vi "Core_Chem_User_Interface_v1.1.vi"() -> ()   [LabVIEW 2014]
uses:
  C:/Program Files (x86)/National Instruments/LabVIEW 2014/examples/Data Communication/Network Streams/Simple Network Streams/support/Network Stream Command.ctl
  <vilib>/dex/Stream Element Allocation Mode.ctl
  <vilib>/Platform/TimedLoop/XDataNode/timing_clust.ctl
  <vilib>/Platform/TimedLoop/XDataNode/nitl_modes.ctl
  <vilib>/Platform/TimedLoop/XDataNode/wakeup.ctl
  <vilib>/Utility/tcp.llb/UDP Multicast Read-Only Open.vi
  <vilib>/platform/TimedLoop/XDataNode/XDataNode.xnode
  <vilib>/Platform/TimedLoop/XDataNode/XDNodeRunTimeDep.lvlib
  <vilib>/FTP/NI_FTP.lvlib
panel:
  in  "Flight Number 2":string
  out "Create folder error out 2":errorcluster
  out "Network to cRIO live status":bool
  out "Create folder error out":errorcluster
  in  "Confirm Flight Number":bool
  out "PRTAFT_UDP_In":string
  out "TWBOZO01":string
  out "CABOZO01":string
  out "TEIOZO01":string
  out "CHTSOO01":string
  out "CHFGGA01":string
  out "AL52CO01":string
  in  "Flight Number":string
  in  "Tab Control":T1(tab)
  out "MFM":dbl(graph)
  out "PRTAFT_DLU":string
  in  "name":string="239.1.4.6"
  in  "Port":u16=50001
  out "FGGA":string
  out "CO":string
  out "Ozone":string
  out "Cabin Ozone":string
  out "Ambient Ozone":string
  out "SO2":string
  out "Raw Signal (Hz)":dbl(graph)
  out "CO Concentration":dbl(graph)
  out "Fluorsecence Cell Pressure":dbl(graph)
  out "Monochromater Flow":dbl(graph)
  out "Lamp Flow Controller":dbl(graph)
  in  "CO UDP Time Offset":i32=1
  out "CO2 Pressure\nDelivery (PSIA)":dbl(slide) scale=0.0..100.0
  out "CO CAL Status":bool
  out "Std\nContent (barG)":dbl(slide) scale=0.0..220.0
  out "N2\nContent (barG)":dbl(slide) scale=0.0..220.0
  out "CO2\nContent (barG)":dbl(slide) scale=0.0..170.0
  in  "CO CAL":bool
  in  "CO Vacuum (eV7)":bool
  out "CO Event error out":errorcluster
  out "CO command sender error out":errorcluster
  out "CO Zero":T2(array[cluster])
  out "CO Sensitivity":T3(array[cluster])
  in  "Ozone V6":bool
  out "TEI49C Sample Flow B":dbl(graph)
  out "TEi49C Concentration":dbl(graph)
  out "TEI49C Sample Flow A":dbl(graph)
  out "Ozone Event error out":errorcluster
  out "Ozone command sender error out":errorcluster
  out "Ozone Zeroing\nTime Remain (sec)":u32
  in  "Ozone Zeroing":bool
  in  "Ozone UDP Time Offset":i32=1
  in  "FGGA Pump":bool
  in  "FGGA Shutdown":bool
  in  "V1":bool
  in  "V2":bool
  in  "MFC_1\nSLPM Value":dbl
  in  "V3":bool
  in  "V4":bool
  in  "FGGA Restart":bool
  out "MFC1 Cal Flow":dbl(graph)
  out "Cell temperature":dbl(graph)
  out "Cell pressure":dbl(graph)
  out "CO2 Dry":dbl(graph)
  out "CH4 Dry":dbl(graph)
  out "H2O":dbl(graph)
  out "CO2":dbl(graph)
  out "CH4":dbl(graph)
  in  "Flush High Tank":bool
  in  "Flush Low Tank":bool
  in  "Flush Target Tank":bool
  out "Flush High Tank\nTime Remain (sec)":u32
  out "Flush Low Tank\nTime Remain (sec)":u32
  out "Flush Target Tank\nTime Remain (sec)":u32
  in  "High Cal":bool
  out "High Cal\nFlush Time Remain (sec)":u32
  out "High Cal\nCal Time Remain (sec)":u32
  in  "Low Cal":bool
  in  "Target Cal":bool
  in  "Span Cal Synchronise with\nCO":bool
  out "Low Cal\nFlush Time Remain (sec)":u32
  out "Low Cal\nCal Time Remain (sec)":u32
  out "Target Cal\nFlush Time Remain (sec)":u32
  out "Target Cal\nCal Time Remain (sec)":u32
  in  "MFC_1 User Set Value":dbl=3.0
  out "FGGA command sender error out":errorcluster
  out "FGGA Event Error out":errorcluster
  in  "FGGA UDP Time Offset":i32=1
  in  "FGGA pump\nsync to WoW":bool
  out "WoW Flag":string="0"
  in  "Inst_alm_thresh":i32=220
  in  "3hr_alm_thresh":i32=80
  in  "Simulate Inst Conc":i32
  in  "Simulate 3hr Average Conc":dbl
  in  "Simulate 2B Conc":bool
  out "2B Ozone concentration":dbl(graph)
  out "2B Ozone flow rate":dbl(graph)
  out "2BOzone Event error out":errorcluster
  out "2BOzone command sender error out":errorcluster
  in  "Ambient = OFF\nCabin = ON":bool
  in  "V9":bool
  in  "V8":bool
  in  "SO2 V6":bool
  in  "MFC_2\nSLPM Value":dbl
  in  "MFC_3\nSLPM Value":dbl=2.0
  in  "Simulate STEL Conc":dbl
  in  "Simulate TWA Conc":dbl
  in  "SO2 Offset":dbl
  in  "SO2 Slope":dbl=1.0
  in  "10mins STEL Limit":i32=700
  in  "8hr TWA Limit":i32=490
  in  "Simulate Conc":bool
  out "TEI43i MFC2 Cal Flow":dbl(graph)
  out "TEI43i MFC3 Sample Flow":dbl(graph)
  out "TEi43C Concentration":dbl(graph)
  out "TEI43C Sample Flow":dbl(graph)
  out "SO2 Event error out":errorcluster
  out "SO2 command sender error out":errorcluster
  in  "SO2 Flush":bool
  in  "SO2 CAL":bool
  in  "MFC_2 User Set Value":dbl=2.5
  in  "MFC_3 User Set Value":dbl=2.0
  out "SO2 Flush\nTime Remain (sec)":u32
  in  "SO2 Zeroing":bool
  out "SO2 Zeroing\nTime Remain (sec)":u32
  out "SO2 CAL\nTime Remain (sec)":u32
  in  "SO2 UDP Time Offset":i32=1
  in  "cRIO File IO Stop\n(USB Flash Drive Unmount)":bool
  in  "FTP ASCII Files to Local":bool
  in  "Transfer FGGA Files":bool
  out "File List":string[](array[string])
  out "FGGA File Transfer Error out":errorcluster
  out "Move to FM Error out":errorcluster
  out "USB Disk Space Used %":dbl(slide) scale=0.0..100.0
  out "PTP Sync":bool
  out "CPU Total %":dbl(graph)
  # "conc\ncounts\nsens\nzero\nlampflow\nlamptemp\nmonoflow\nmonotemp\nmonopress\ncellpress\ncalpress\ntemppmt\ncalconc\nerr\ncal_counter\nerr_counter\nCO_vacuum_status\nIn_Cal\nALEG1_press_delivery\nALREG1_press_content\nALREG2_press_content\nALREG3_press_content"
  # "concentration\npmt_volt\nlamp_volt\nlamp_intens\ninternal_temper\nreact_temper\nreact_press\nflow\nflags\nten_min_so2\neight_hr_so2\nten_min_so2_alm\neight_hr_so2_alm\nMFC_2absolute_pressure\nMFC_2temperature\nMFC_2volumetic_flow\nMFC_2mass_flow\nMFC_2set_point\nMFC_3_absolute_pressure\nMFC_3_temperature\nMFC_3volumetic_flow\nMFC_3mass_flow\nMFC_3set_point\nV6\nV8\nV9\nMFC2_Set_Value\nMFC3_Set_Value"
  # "ch4\nco2\nh2o\npress_torr\ntemp_c\nfit_flag\nrda_usec\nrdb_usec\nch4_dry\nco2_dry\nMFC_1_absolute_pressure\nMFC_1_temperature\nMFC_1volumetic_flow\nMFC_1mass_flow\nMFC_1set_point\nV1\nV2\nV3\nV4\nrestart_FGGA\nFGGA_Pump\nCAL_MFC_1Set_Value"
  # "conc\ntemp\npress\nflow"
  # "conc\ntemp\npress\nflow\nthreehr_oz\nInst_alarm\nthreehr_alarm"
  # "conc\nbenchtemp\npress\ncellAint\ncellBint\nFlowA\nFlowB\nlamptemp\nflag\nV6"
  # "DIRECT CONTROL"
  # "DIRECT CONTROLS"
  # "DIRECT CONTROLS"
  # "TEi43c"
  # "TEi43i"
  # "DIRECT CONTROLS"
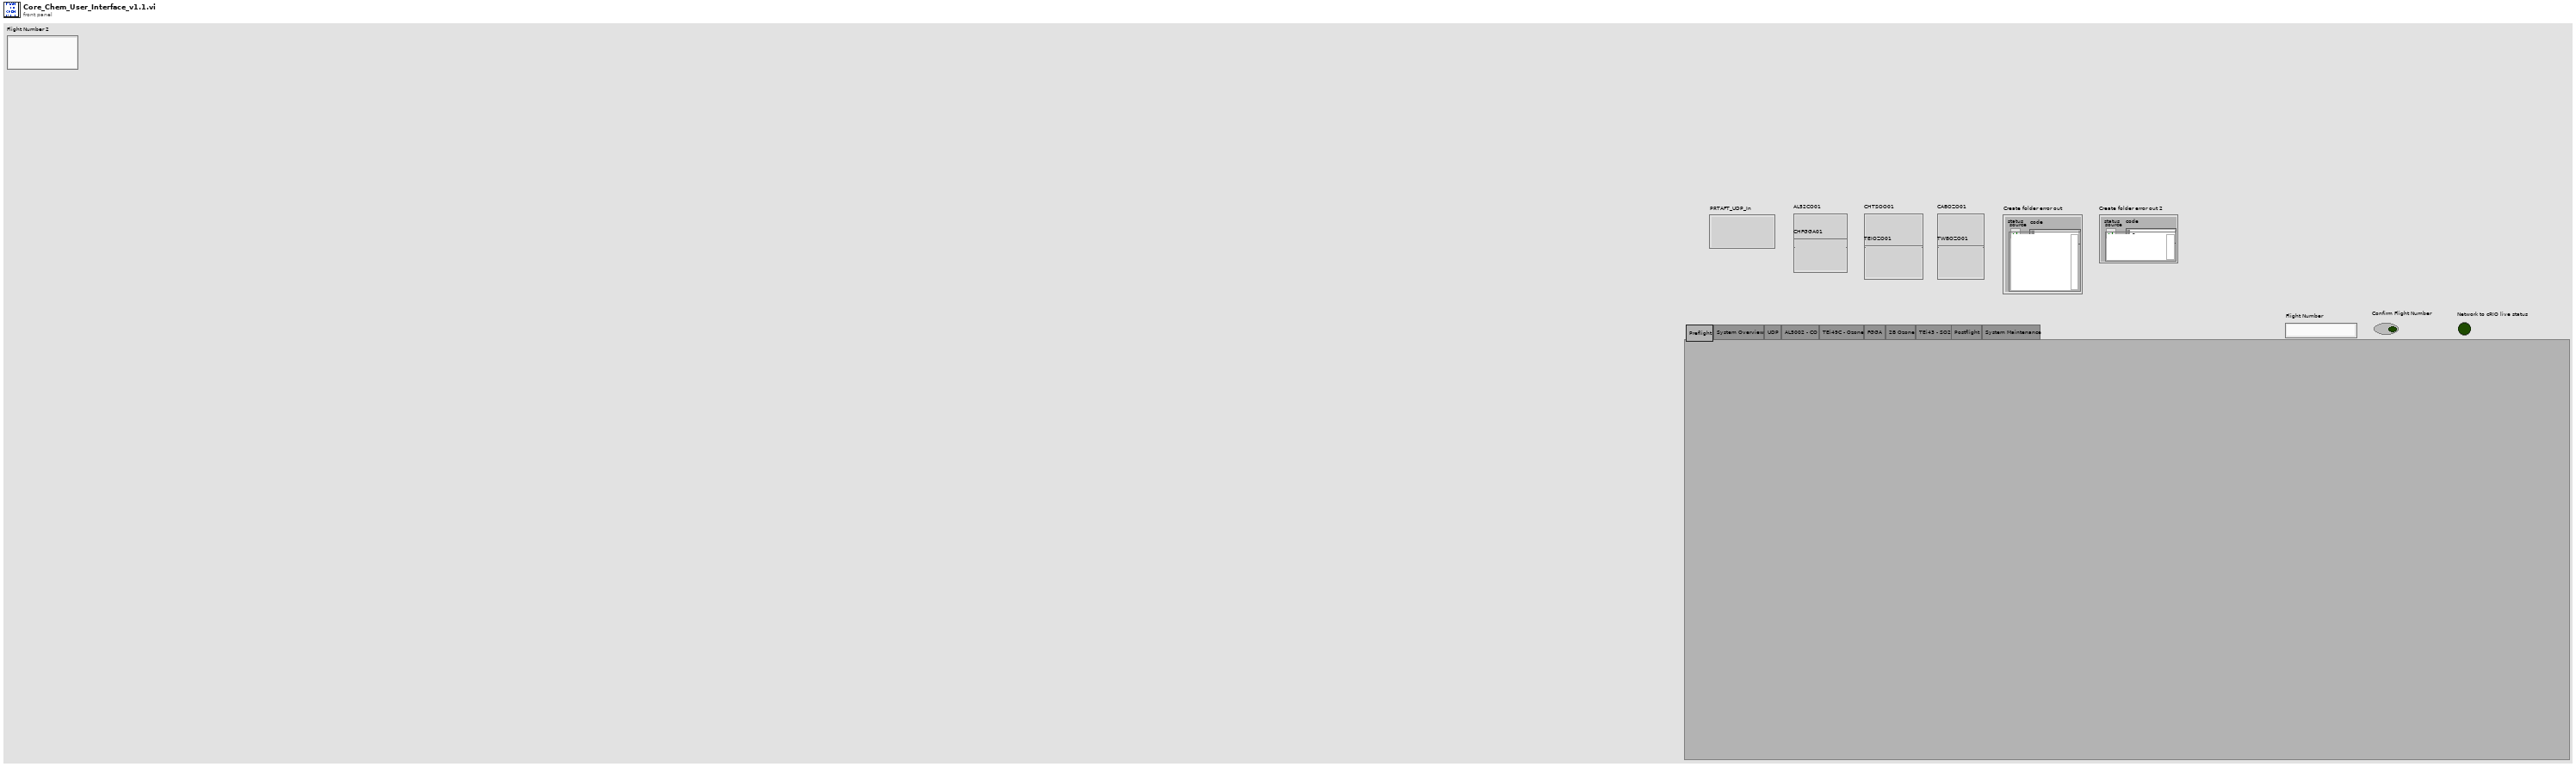
[diagram p1: front panel]
types:
  T1 = enum32{"Preflight", "System Overview", "UDP", "AL5002 - CO", "TEi49C - Ozone", "FGGA", "2B Ozone", "TEi43 - SO2", "Postflight", "System Maintenance"}
  T2 = cluster{"time stamp":timestamp, "CO Offset":dbl}[]
  T3 = cluster{"time stamp":timestamp, "CO Sensitivity":dbl}[]
  T4 = typedef "Network Stream Command.ctl" = cluster{"Message":string, "Message Data":variant}
  T5 = typedef "Stream Element Allocation Mode.ctl" = u32
  T6 = typedef "XDNodeRunTimeDep.lvlib/timing_clust.ctl" = cluster{"Expected End [f-1]":u64, "Actual End [f-1]":u64, "Finished Late? [f-1]":bool, "Expected End [i-1]":u64, "Actual End [i-1]":u64, "Finished Late? [i-1]":bool, "Expected Start [i]":u64, "Actual Start [i]":u64, "Expected Start [f]":u64, "Actual Start [f]":u64, "Source Name":string, "Structure Name":string, "Period":i64, "Deadline":i64, "Offset":i64, "Start":i64, "Priority":i32, "Timeout":i32, "Mode":T7, "Wakeup Reason":T8, "Error":errorcluster, "Source Type":string, "Secondary Source Type":string, "Global End Time":u64, "Global Start Time":u64, "Frame Duration":u64, "Iteration Duration":u64, "Assigned CPU":i32, "I/O Scan Engine Mode":u32}
  T7 = typedef "XDNodeRunTimeDep.lvlib/nitl_modes.ctl" = enum32{"No Change", "Process missed periods, maintain original phase", "Discard missed periods, maintain original phase", "Process missed periods, ignore original phase", "Discard missed periods, ignore original phase"}
  T8 = typedef "XDNodeRunTimeDep.lvlib/wakeup.ctl" = enum32{"Normal", "Aborted", "Asynchronous wakeup", "Timing source error", "Timed loop error", "Timeout"}
  T9 = typedef "NI_FTP.lvlib/FTP Session.ctl" = refnum<k5>
  T10 = typedef "NI_FTP.lvlib/FTP File Info.ctl" = cluster{"type":enum16{"unknown", "file", "dir", "link"}, "permissions":string, "owner":string, "group":string, "size":i32, "date":string, "name":string, "link name":string}
  T11 = cluster{"Message":string, "Message 2":string, "Message 3":string}
  T12 = cluster{"Message":string, "Message 2":string, "Message 3":string, "Message 4":string}
  T13 = cluster{"Message":string, "Message 3":string, "Message 4":string}
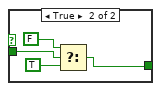
[diagram p8: hidden frame]
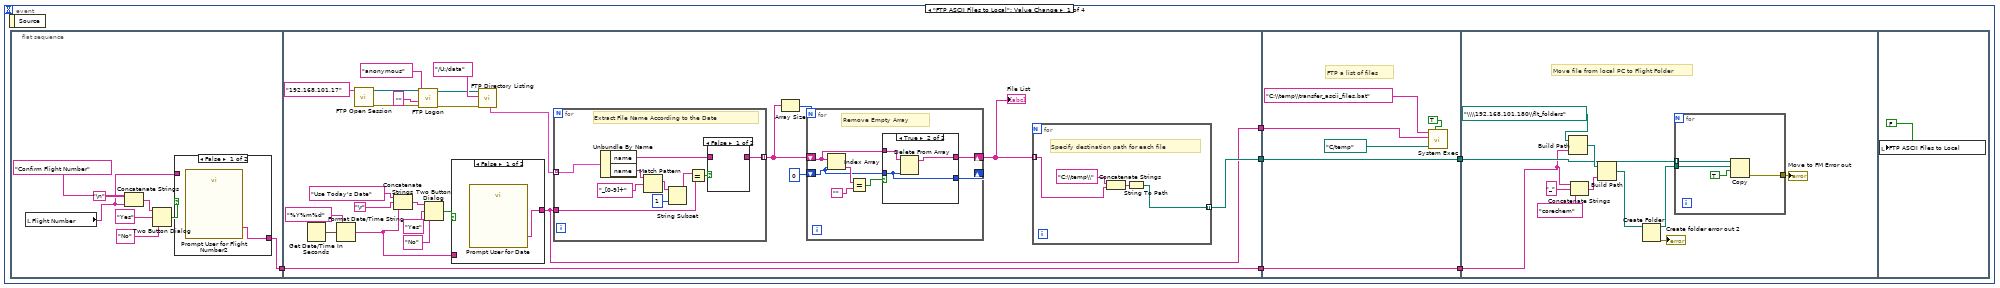
[diagram p11: hidden frame]
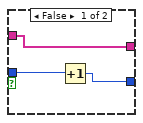
[diagram p14: hidden frame]
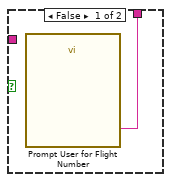
[diagram p16: hidden frame]
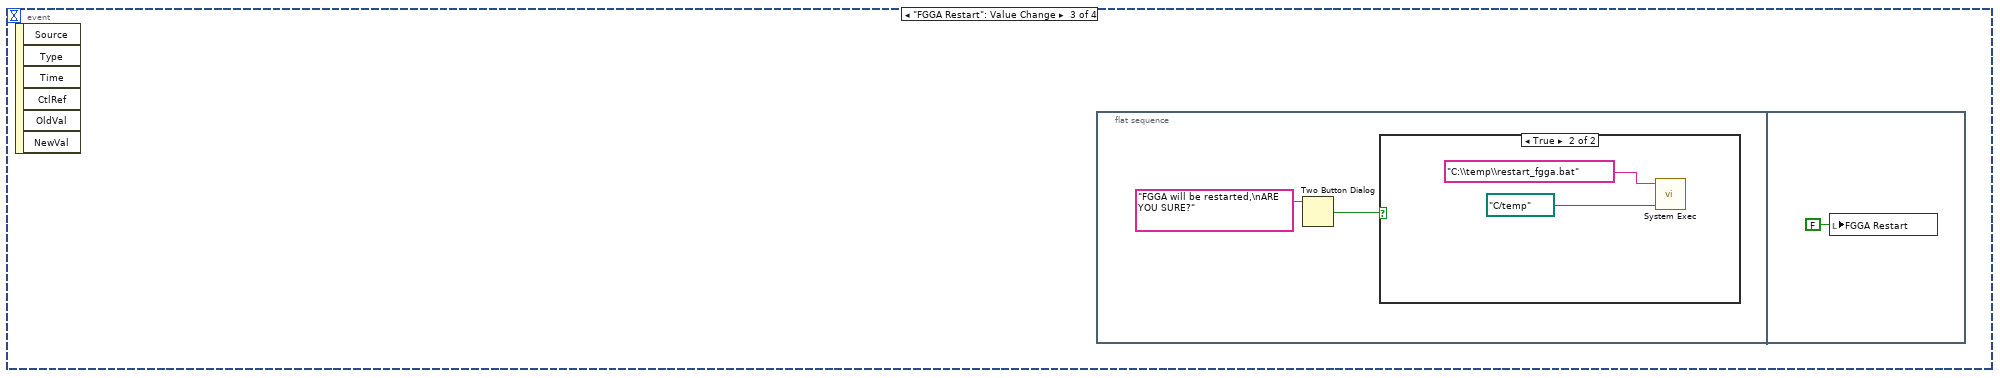
[diagram p18: hidden frame]
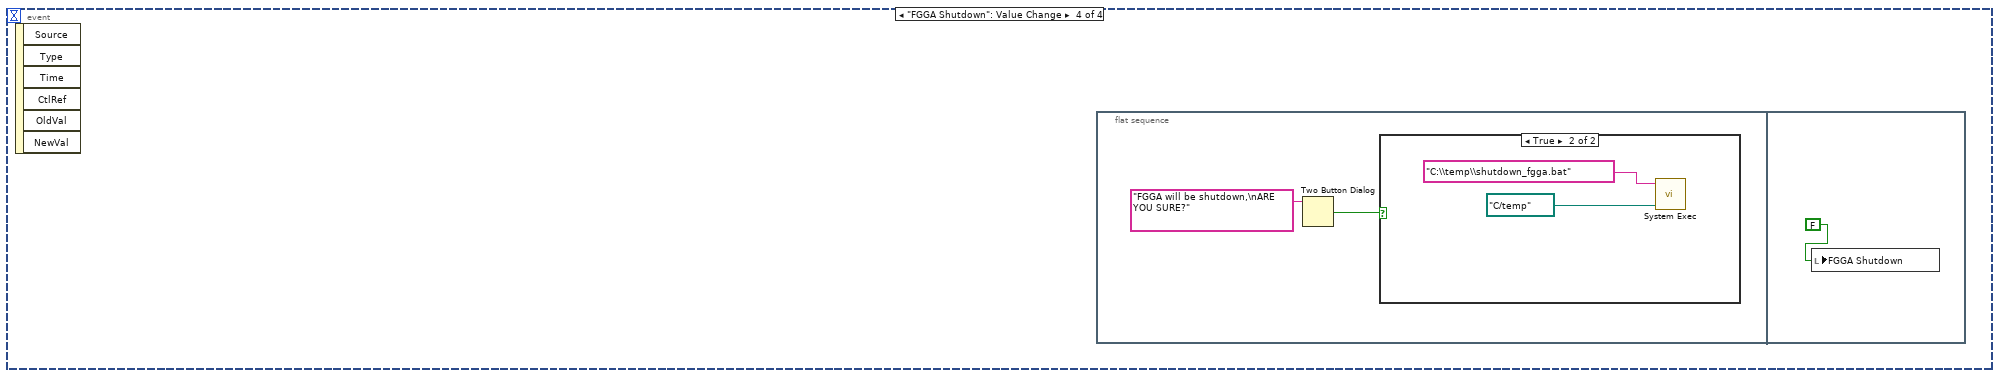
[diagram p20: hidden frame]
diagram:
  w4 = "XXXX"
  w7 = 0
  w8 = 0.0
  w14 = T4 {"Message"="", "Message Data"=variant} ("Message Cluster")
  w20 = T5 0 items=["allocate as needed", "pre-allocate"] ("element allocation mode")
  w26 = T4 {"Message"="", "Message Data"=variant} ("Message Cluster")
  w32 = T5 0 items=["allocate as needed", "pre-allocate"] ("element allocation mode")
  w37 = T4 {"Message"="", "Message Data"=variant} ("Message Cluster")
  w43 = T5 0 items=["allocate as needed", "pre-allocate"] ("element allocation mode")
  w53 = T5 0 items=["allocate as needed", "pre-allocate"] ("element allocation mode")
  w55 = T4 {"Message"="", "Message Data"=variant} ("Message Cluster")
  w62 = T5 0 items=["allocate as needed", "pre-allocate"] ("element allocation mode")
  w64 = T4 {"Message"="", "Message Data"=variant} ("Message Cluster")
  n1 = local write "cRIO File IO Stop\n(USB Flash Drive Unmount)"(FALSE ("Stop File Write")) -> ()
  n2 = local write "Flight Number"(w4) -> ()
  n3 = while {
    shift-right: [w68] -> _
    shift-left: w4 -> [w67]
    stop <- FALSE stop-if-true
    n4 = Not Equal?(x=w67, y="Flight Number") -> (x != y?=w70:bool)
    n5 = case shown="True" w70 {
      tunnel: [w73 w74] -> w68
      tunnel: "Flight Number" -> [_ w74]
      tunnel: w67 -> [w73 _]
      frame False {
      }
      frame True {
        n6 = One Button Dialog(message="Flight Number changed,\nPress flight number button to confirm") -> ()  [unwired: 1 in, 1 out]
      }
    }
    n7 = Wait (ms)(milliseconds to wait=u32 1000) -> ()  [unwired: 1 out]
  }
  n8 = while {
    stop <- FALSE stop-if-true
    # "UDP Read"
    n9 = String To IP(1:"name") -> (0:w81:u32)
    n10 = call-poly <vilib>:"UDP Multicast Open.vi"("multicast addr"=w81, "port"="Port") -> ("error out"=w79:errorcluster, "connection ID"=w78:refnum<k16>)  [unwired: 7 in, 1 out]
    n11 = Wait (ms)(milliseconds to wait=u32 1000) -> ()  [unwired: 1 out]
    n12 = case shown="No Error" w79 {
      selector: w79 -> [w85 _]
      tunnel: w78 -> [w84 _]
      frame No Error {
        w83 = ""
        n13 = while {
          tunnel: w85 -> [w131]
          tunnel: w84 -> [w130]
          shift-right: [w126] -> _
          shift-left: w83 -> [w127]
          shift-right: [w117] -> _
          shift-left: w83 -> [w119]
          shift-right: [w111] -> _
          shift-left: w83 -> [w113]
          shift-right: [w105] -> _
          shift-left: w83 -> [w106]
          shift-right: [w99] -> _
          shift-left: w83 -> [w100]
          shift-right: [w93] -> _
          shift-left: w83 -> [w94]
          shift-right: [w88] -> _
          shift-left: w83 -> [w89]
          stop <- w129 stop-if-true
          n14 = UDP Read(connection ID=w130, 8:w131) -> (data out=w86:string, error out=w129:errorcluster)  [unwired: 2 in, 3 out]
          n15 = Match Pattern(string=w86, regular expression="$TEIOZO01,") -> (match substring=w125:string, after substring=w124:string)  [unwired: 1 in, 2 out]
          n16 = Match Pattern(string=w86, regular expression="$TWBOZO01,") -> (match substring=w103:string, after substring=w102:string)  [unwired: 1 in, 2 out]
          n17 = Match Pattern(string=w86, regular expression="$CABOZO01,") -> (match substring=w109:string, after substring=w108:string)  [unwired: 1 in, 2 out]
          n18 = Match Pattern(string=w86, regular expression="$CHTSOO01,") -> (match substring=w97:string, after substring=w96:string)  [unwired: 1 in, 2 out]
          n19 = Match Pattern(string=w86, regular expression="$CHFGGA01,") -> (match substring=w121:string, after substring=w120:string)  [unwired: 1 in, 2 out]
          n20 = Match Pattern(string=w86, regular expression="$AL52CO01,") -> (match substring=w115:string, after substring=w114:string)  [unwired: 1 in, 2 out]
          n21 = Match Pattern(string=w86, regular expression="$PRTAFT01,") -> (match substring=w92:string, after substring=w91:string)  [unwired: 1 in, 2 out]
          n22 = Concatenate Strings(w125, w124) -> (w123:string)
          n23 = Concatenate Strings(w103, w102) -> (w101:string)
          n24 = Concatenate Strings(w109, w108) -> (w107:string)
          n25 = Concatenate Strings(w97, w96) -> (w95:string)
          n26 = Concatenate Strings(w121, w120) -> (w118:string)
          n27 = Concatenate Strings(w115, w114) -> (w112:string)
          n28 = Concatenate Strings(w92, w91) -> (w87:string)
          n29 = Replace Substring(4:w101, 5:w100) -> (1:w99:string)  [unwired: 2 in, 1 out]
          "TWBOZO01" <- w99
          n30 = Replace Substring(4:w123, 5:w127) -> (1:w126:string)  [unwired: 2 in, 1 out]
          "TEIOZO01" <- w126
          n31 = Replace Substring(4:w107, 5:w106) -> (1:w105:string)  [unwired: 2 in, 1 out]
          "CABOZO01" <- w105
          n32 = Replace Substring(4:w95, 5:w94) -> (1:w93:string)  [unwired: 2 in, 1 out]
          "CHTSOO01" <- w93
          n33 = Replace Substring(4:w87, 5:w89) -> (1:w88:string)  [unwired: 2 in, 1 out]
          "PRTAFT_UDP_In" <- w88
          n34 = Replace Substring(4:w112, 5:w113) -> (1:w111:string)  [unwired: 2 in, 1 out]
          "AL52CO01" <- w111
          n35 = Replace Substring(4:w118, 5:w119) -> (1:w117:string)  [unwired: 2 in, 1 out]
          "CHFGGA01" <- w117
        }
      }
      frame Error {
      }
    }
  }
  n36 = Obtain Queue(name (unnamed)="CO_Command", element data type=w64) -> (queue out=w13:refnum<queue>, error out=w58:errorcluster)  [unwired: 3 in, 1 out]
  n37 = Create Network Stream Writer Endpoint(6:w62, 7:10 ("writer buffer size"), 9:w64, 10:"//192.168.101.17/command/reader/CO" ("reader url"), 11:"/command/writer/CO" ("writer name")) -> (0:w61:errorcluster, 3:w60:refnum<k21>)  [unwired: 2 in]
  n38 = while {
    tunnel: w13 -> [w135]
    tunnel: w58 -> [w134]
    tunnel: [w132] -> _
    stop <- FALSE stop-if-true
    # "CO UI Event Handler Loop"
    n39 = event shown="[4] \"Confirm Flight Number\": Value Change" {
      selector: _ -> [_ _ _ _ _]
      dyn-events: _ -> [_ _ _ _ _]
      timeout: _ -> [_ _ _ _ _]
      tunnel: w135 -> [w142 w149 w153 w160 w167]
      tunnel: w134 -> [w141 w148 w152 w159 w166]
      tunnel: [w136 w143 w151 w158 w165] -> w132
      event "CO CAL": Value Change {
        n40 = event-data() -> ("NewVal"=w139:bool)  [unwired: 1 in]
        n41 = Bundle(cluster=T4 {"Message"="", "Message Data"=variant} ("Message Cluster"), "Message"="CO CAL", "Message Data"=w139) -> (w137:T4)
        n42 = Enqueue Element(queue=w142, element=w137, error in (no error)=w141) -> (error out=w136:errorcluster)  [unwired: 1 in, 2 out]
      }
      event "CO UDP Time Offset": Value Change {
        n43 = event-data() -> ("NewVal"=w146:i32)  [unwired: 1 in]
        n44 = Bundle(cluster=T4 {"Message"="", "Message Data"=variant} ("Message Cluster"), "Message"="UDP Time Offset", "Message Data"=w146) -> (w144:T4)
        n45 = Enqueue Element(queue=w149, element=w144, error in (no error)=w148) -> (error out=w143:errorcluster)  [unwired: 1 in, 2 out]
      }
      event "CO Vacuum (eV7)": Value Change {
        n46 = event-data() -> ("NewVal"=w150:bool)  [unwired: 1 in]
        n47 = Bundle(cluster=T4 {"Message"="", "Message Data"=variant} ("Message Cluster"), "Message"="CO Vacuum", "Message Data"=w150) -> (w154:T4)
        n48 = Enqueue Element(queue=w153, element=w154, error in (no error)=w152) -> (error out=w151:errorcluster)  [unwired: 1 in, 2 out]
      }
      event "cRIO File IO Stop\n(USB Flash Drive Unmount)": Value Change {
        n49 = event-data() -> ("NewVal"=w157:bool)  [unwired: 1 in]
        n50 = Bundle(cluster=T4 {"Message"="", "Message Data"=variant} ("Message Cluster"), "Message"="Stop File Write", "Message Data"=w157) -> (w161:T4)
        n51 = Enqueue Element(queue=w160, element=w161, error in (no error)=w159) -> (error out=w158:errorcluster)  [unwired: 1 in, 2 out]
      }
      event "Confirm Flight Number": Value Change {
        n52 = event-data() -> ()  [unwired: 1 in, 1 out]
        n53 = local read "Flight Number"() -> (w164:string)
        n54 = Bundle(cluster=T4 {"Message"="", "Message Data"=variant} ("Message Cluster"), "Message"="Flight Number", "Message Data"=w164) -> (w168:T4)
        n55 = Enqueue Element(queue=w167, element=w168, error in (no error)=w166) -> (error out=w165:errorcluster)  [unwired: 1 in, 2 out]
      }
    }
    "CO Event error out" <- w132
  }
  n56 = while {
    tunnel: w13 -> [w178]
    shift-right: [w173] -> _
    shift-left: w60 -> [w175]
    shift-right: [w171] -> w49
    shift-left: w61 -> [w177]
    tunnel: w58 -> [w172]
    stop <- w171 stop-if-true
    # "CO UI Command Sender"
    n57 = Dequeue Element(queue=w178, error in (no error)=w172) -> (element=w174:T4)  [unwired: 1 in, 3 out]
    n58 = Unbundle By Name(w174) -> ("Message"=w176:string)
    n59 = case shown="\"UDP Time Offset\"" w176 {
      tunnel: w177 -> [w179 w183 w190 w197 w204 w211]
      tunnel: w175 -> [w180 w186 w193 w200 w207 w214]
      tunnel: w174 -> [_ w185 w192 w199 w206 w213]
      tunnel: [w179 w182 w189 w196 w203 w210] -> w171
      tunnel: [w180 w181 w188 w195 w202 w209] -> w173
      frame "False", Default {
      }
      frame "CO CAL" {
        n60 = shared-variable-write(w186, w183, w185) -> (w184:refnum<k21>, w187:errorcluster)  [unwired: 1 in, 1 out]
        n61 = Flush Stream(8:w187, 11:w184) -> (0:w182:errorcluster, 3:w181:refnum<k21>)  [unwired: 2 in, 1 out]
      }
      frame "UDP Time Offset" {
        n62 = shared-variable-write(w193, w190, w192) -> (w191:refnum<k21>, w194:errorcluster)  [unwired: 1 in, 1 out]
        n63 = Flush Stream(8:w194, 11:w191) -> (0:w189:errorcluster, 3:w188:refnum<k21>)  [unwired: 2 in, 1 out]
      }
      frame "Stop File Write" {
        n64 = shared-variable-write(w200, w197, w199) -> (w198:refnum<k21>, w201:errorcluster)  [unwired: 1 in, 1 out]
        n65 = Flush Stream(8:w201, 11:w198) -> (0:w196:errorcluster, 3:w195:refnum<k21>)  [unwired: 2 in, 1 out]
      }
      frame "Flight Number" {
        n66 = shared-variable-write(w207, w204, w206) -> (w205:refnum<k21>, w208:errorcluster)  [unwired: 1 in, 1 out]
        n67 = Flush Stream(8:w208, 11:w205) -> (0:w203:errorcluster, 3:w202:refnum<k21>)  [unwired: 2 in, 1 out]
      }
      frame "CO Vacuum" {
        n68 = shared-variable-write(w214, w211, w213) -> (w212:refnum<k21>, w215:errorcluster)  [unwired: 1 in, 1 out]
        n69 = Flush Stream(8:w215, 11:w212) -> (0:w210:errorcluster, 3:w209:refnum<k21>)  [unwired: 2 in, 1 out]
      }
    }
  }
  "CO command sender error out" <- w49
  n70 = node-c288() -> (w12:T6)  [unwired: 4 in]
  n71 = Initialize Array(cluster{"time stamp":timestamp, "Y":dbl} {"time stamp"=timestamp(0 s since 1904-01-01), "Y"=0.0}, 30 ("dimension size")) -> (w9:cluster{"time stamp":timestamp, "Y":dbl}[])
  n72 = timed-loop {
    timing: w12 -> [_]
    timing-out: [_] -> w11
    stop <- _ stop-if-true
    # "PC Tasks"
    n73 = node-c288() -> ()  [unwired: 1 in, 1 out]
    n74 = event shown="[1] \"Transfer FGGA Files\": Value Change" {
      selector: _ -> [_ _ _ _]
      dyn-events: _ -> [_ _ _ _]
      timeout: _ -> [_ _ _ _]
      event "FTP ASCII Files to Local": Value Change {
        n75 = event-data() -> ()  [unwired: 1 in, 1 out]
        n76 = flat-sequence {
          tunnel: [w224] -> w218
          tunnel: [w236] -> w223
          tunnel: [w235] -> w221
          tunnel: [w234] -> w219
          tunnel: w218 -> [w234]
          tunnel: w223 -> [w294]
          tunnel: [w294] -> w222
          tunnel: w221 -> [w290]
          tunnel: [w289] -> w220
          tunnel: w219 -> [w289]
          tunnel: w222 -> [w300]
          tunnel: w220 -> [w295]
          frame #0 {
            n77 = local read "Flight Number"() -> (w225:string)
            n78 = Concatenate Strings("Confirm Flight Number" ("message"), "\n", w225) -> (w230:string)
            n79 = Two Button Dialog(message=w230, 1:"No" ("F button name (\"Cancel\")"), 2:"Yes" ("T button name (\"OK\")")) -> (T button?=w226:bool)
            n80 = case shown="False" w226 {
              tunnel: w225 -> [_ w233]
              tunnel: [w232 w233] -> w224
              frame False {
                n81 = call "Prompt User for Flight Number2"() -> ("Flight Number BXXX"=w232:string)  [unwired: 17 in, 2 out]
              }
              frame True {
              }
            }
          }
          frame #1 {
            n82 = Get Date/Time In Seconds() -> (seconds since 1Jan1904=w240:timestamp)
            n83 = Format Date/Time String(time format string (%c)="%Y%m%d", seconds (now)=w240) -> (date/time string=w238:string)  [unwired: 1 in]
            n84 = call <vilib>:"FTP Open Session.vi"("address"="192.168.101.17") -> ("error out"=w255:errorcluster, "ftp session"=w256:T9)  [unwired: 7 in, 2 out]
            n85 = Concatenate Strings("Use Today's Date" ("message"), "\r", w238) -> (w244:string)
            n86 = call <vilib>:"FTP Logon.vi"("error in (no error)"=w255, "password"="", "user"="anonymous", "ftp session"=w256) -> ("error out"=w252:errorcluster, "ftp session out"=w251:T9)  [unwired: 4 in, 2 out]
            n87 = Two Button Dialog(message=w244, 1:"No" ("F button name (\"Cancel\")"), 2:"Yes" ("T button name (\"OK\")")) -> (T button?=w241:bool)
            n88 = case shown="False" w241 {
              tunnel: [w259 w260] -> w235
              tunnel: w238 -> [_ w260]
              frame False {
                n89 = call "Prompt User for Date"() -> ("Date"=w259:string)  [unwired: 17 in, 2 out]
              }
              frame True {
              }
            }
            n90 = call <vilib>:"FTP Directory Listing.vi"("error in (no error)"=w252, "directory path"="/U:/data", "ftp session"=w251) -> ("dir list"=w250:T10[])  [unwired: 4 in, 4 out]
            n91 = for {
              tunnel: w250 -> [w280] mode=indexing
              tunnel: [w279] -> w247 mode=indexing
              tunnel: w235 -> [w278]
              # "Extract File Name According to the Date"
              n92 = Unbundle By Name(w280) -> ("name"=w286:string, "name"=w285:string)
              n93 = Match Pattern(string=w285, regular expression="_[0-9]+") -> (match substring=w283:string)  [unwired: 1 in, 3 out]
              n94 = String Subset(string=w283, offset (0)=1) -> (substring=w281:string)  [unwired: 1 in]
              n95 = Equal?(x=w281, y=w278) -> (x = y?=w287:bool)
              n96 = case shown="False" w287 {
                tunnel: w286 -> [_ w288]
                tunnel: [_ w288] -> w279
                frame False {
                }
                frame True {
                }
              }
            }
            n97 = Array Size(array=w247) -> (size(s)=w249:i32)
            n98 = for {
              N: w249 -> [_]
              shift-right: [w267] -> w237
              shift-left: w247 -> [w268]
              shift-right: [w265] -> _
              shift-left: 0 -> [w266]
              # "Remove Empty Array"
              n99 = Index Array(array=w268, index=w266) -> (element=w270:string)
              n100 = Equal?(x=w270, y="") -> (x = y?=w269:bool)
              n101 = case shown="True" w269 {
                tunnel: w268 -> [w274 w277]
                tunnel: w266 -> [w273 w275]
                tunnel: [w274 w276] -> w267
                tunnel: [w272 w275] -> w265
                frame False {
                  n102 = Increment(x=w273) -> (x+1=w272:i32)
                }
                frame True {
                  n103 = Delete From Array(array=w277, index=w275) -> (array with subset deleted=w276:string[])  [unwired: 1 in, 1 out]
                }
              }
            }
            "File List" <- w237
            n104 = for {
              tunnel: w237 -> [w263] mode=indexing
              tunnel: [w261] -> w236 mode=indexing
              # "Specify destination path for each file"
              n105 = Concatenate Strings("C:\\temp\\", w263) -> (w262:string)
              n106 = String To Path(string=w262) -> (path=w261:path)
            }
          }
          frame #2 {
            # "FTP a list of files"
            n107 = call <vilib>:"System Exec.vi"("wait until completion? (T)"=TRUE, "working directory"=path "C:/temp", "standard input"=w290, "command line"="C:\\temp\\transfer_ascii_files.bat") -> ()  [unwired: 4 in, 4 out]
          }
          frame #3 {
            # "Move file from local PC to Flight Folder"
            n108 = Build Path(base path=path "\\\\192.168.101.180\\flt_folders" ("path"), name or relative path=w295) -> (appended path=w302:path)
            n109 = Concatenate Strings(w295, "_" ("string"), "corechem" ("string")) -> (w301:string)
            n110 = Build Path(base path=w302, name or relative path=w301) -> (appended path=w297:path)
            n111 = Create Folder(path (use dialog)=w297) -> (created path=w296:path, error out=→"Create folder error out 2":errorcluster)  [unwired: 2 in, 1 out]
            n112 = for {
              tunnel: w296 -> [w309]
              tunnel: [w308] -> w299
              tunnel: w300 -> [w306] mode=indexing
              n113 = Copy(9:TRUE ("overwrite (F)"), 10:w309, 11:w306) -> (0:w308:errorcluster)  [unwired: 2 in, 2 out]
            }
            "Move to FM Error out" <- w299
          }
          frame #4 {
            n114 = local write "FTP ASCII Files to Local"(FALSE ("FTP Files to Local")) -> ()
          }
        }
      }
      event "Transfer FGGA Files": Value Change {
        n115 = event-data() -> ()  [unwired: 1 in, 6 out]
        n116 = flat-sequence {
          tunnel: [w315] -> w314
          tunnel: w314 -> [w327]
          tunnel: [w327] -> w313
          tunnel: [w326] -> w312
          tunnel: [w325] -> w311
          tunnel: w313 -> [w343]
          tunnel: w312 -> [w345]
          tunnel: w311 -> [w344]
          frame #0 {
            n117 = local read "Flight Number"() -> (w316:string)
            n118 = Concatenate Strings("Confirm Flight Number" ("message"), "\n", w316) -> (w318:string)
            n119 = Two Button Dialog(message=w318, 1:"No" ("F button name (\"Cancel\")"), 2:"Yes" ("T button name (\"OK\")")) -> (T button?=w322:bool)
            n120 = case shown="True" w322 {
              tunnel: w316 -> [_ w324]
              tunnel: [w323 w324] -> w315
              frame False {
                n121 = call "Prompt User for Flight Number"() -> ("Flight Number BXXX"=w323:string)  [unwired: 17 in, 2 out]
              }
              frame True {
              }
            }
          }
          frame #1 {
            n122 = Two Button Dialog(message="Get FGGA Files\nof Today's Date?", 1:"No" ("F button name (\"Cancel\")"), 2:"Yes" ("T button name (\"OK\")")) -> (T button?=w331:bool)
            n123 = case shown="False" w331 {
              selector: w331 -> [w333 w334]
              tunnel: [w333 w334] -> w325
              tunnel: [w332 _] -> w326
              frame False {
                n124 = call "Prompt User for Date"() -> ("Date"=w332:string)  [unwired: 17 in, 2 out]
              }
              frame True {
              }
            }
          }
          frame #2 {
            n125 = Build Path(base path=path "\\\\192.168.101.180\\flt_folders" ("path"), name or relative path=w343) -> (appended path=w337:path)
            n126 = Concatenate Strings(w343, "_" ("string"), "corechem" ("string")) -> (w336:string)
            n127 = Build Path(base path=w337, name or relative path=w336) -> (appended path=w342:path)
            n128 = Create Folder(path (use dialog)=w342) -> (error out=→"Create folder error out":errorcluster)  [unwired: 2 in, 2 out]
            n129 = call "FGGA_files_transfer.vi"("Flight_num"=w343, "Get current?"=w344, "Date"=w345, "Flight Folder Path"=w342) -> ("error IO"=→"FGGA File Transfer Error out":errorcluster)  [unwired: 11 in]
          }
          frame #3 {
            n130 = local write "Transfer FGGA Files"(FALSE) -> ()
          }
        }
      }
      event "FGGA Restart": Value Change {
        n131 = event-data() -> ()  [unwired: 1 in, 6 out]
        n132 = flat-sequence {
          frame #0 {
            n133 = Two Button Dialog(message="FGGA will be restarted,\nARE YOU SURE?") -> (T button?=w348:bool)  [unwired: 2 in]
            n134 = case shown="True" w348 {
              frame False {
              }
              frame True {
                n135 = call <vilib>:"System Exec.vi"("working directory"=path "C:/temp", "command line"="C:\\temp\\restart_fgga.bat") -> ()  [unwired: 6 in, 4 out]
              }
            }
          }
          frame #1 {
            n136 = local write "FGGA Restart"(FALSE ("FGGA Restart")) -> ()
          }
        }
      }
      event "FGGA Shutdown": Value Change {
        n137 = event-data() -> ()  [unwired: 1 in, 6 out]
        n138 = flat-sequence {
          frame #0 {
            n139 = Two Button Dialog(message="FGGA will be shutdown,\nARE YOU SURE?") -> (T button?=w353:bool)  [unwired: 2 in]
            n140 = case shown="True" w353 {
              frame False {
              }
              frame True {
                n141 = call <vilib>:"System Exec.vi"("working directory"=path "C:/temp", "command line"="C:\\temp\\shutdown_fgga.bat") -> ()  [unwired: 6 in, 4 out]
              }
            }
          }
          frame #1 {
            n142 = local write "FGGA Shutdown"(FALSE ("FGGA Restart")) -> ()
          }
        }
      }
    }
    n143 = node-c288() -> ()  [unwired: 1 in, 1 out]
  }
  n144 = while {
    shift-right: [w440] -> _
    shift-left: w8 -> [w438]
    shift-right: [w442] -> _
    shift-left: w7 -> [w443]
    shift-right: [w441] -> _
    shift-left: w9 -> [w445]
    shift-right: [w433] -> _
    shift-left: w9 -> [w435]
    shift-right: [w430] -> _
    shift-left: w8 -> [w429]
    shift-right: [w432] -> _
    shift-left: w7 -> [w434]
    shift-right: [w425] -> _
    shift-left: FALSE -> [w426]
    stop <- FALSE stop-if-true
    w371 = ""
    w363 = "%s" ("format string")
    w564 = "%s" ("format string")
    w569 = "%s" ("format string")
    w574 = "%s" ("format string")
    w580 = "%s" ("format string")
    w586 = "%s" ("format string")
    w590 = "%s" ("format string")
    # "UDP Data Processing"
    n145 = local read "CHFGGA01"() -> (w593:string)
    n146 = local read "TWBOZO01"() -> (w568:string)
    n147 = local read "AL52CO01"() -> (w585:string)
    n148 = local read "CABOZO01"() -> (w573:string)
    n149 = local read "TEIOZO01"() -> (w579:string)
    n150 = local read "CHTSOO01"() -> (w563:string)
    n151 = local read "PRTAFT_UDP_In"() -> (w374:string)
    n152 = local read "Ambient = OFF\nCabin = ON"() -> (w467:bool)
    n153 = Spreadsheet String To Array(delimiter (Tab)=",", format string=w590, spreadsheet string=w593, array type (2D Dbl)=string[] []) -> (array=w540:string[])
    n154 = Spreadsheet String To Array(delimiter (Tab)=",", format string=w586, spreadsheet string=w585, array type (2D Dbl)=string[] []) -> (array=w561:string[])
    n155 = Spreadsheet String To Array(delimiter (Tab)=",", format string=w574, spreadsheet string=w573, array type (2D Dbl)=string[] []) -> (array=w464:string[])
    n156 = Spreadsheet String To Array(delimiter (Tab)=",", format string=w580, spreadsheet string=w579, array type (2D Dbl)=string[] []) -> (array=w538:string[])
    n157 = Spreadsheet String To Array(delimiter (Tab)=",", format string=w569, spreadsheet string=w568, array type (2D Dbl)=string[] []) -> (array=w463:string[])
    n158 = Spreadsheet String To Array(delimiter (Tab)=",", format string=w564, spreadsheet string=w563, array type (2D Dbl)=string[] []) -> (array=w536:string[])
    n159 = Array To Spreadsheet String(delimiter (Tab)="\r", array=w540, 3:w590) -> (spreadsheet string=→"FGGA":string)
    n160 = Spreadsheet String To Array(delimiter (Tab)=",", format string=w363, spreadsheet string=w374, array type (2D Dbl)=string[] []) -> (array=w362:string[])
    n161 = Array To Spreadsheet String(delimiter (Tab)="\r", array=w561, 3:w586) -> (spreadsheet string=→"CO":string)
    n162 = Array To Spreadsheet String(delimiter (Tab)="\r", array=w464, 3:w574) -> (spreadsheet string=→"Cabin Ozone":string)
    n163 = Array To Spreadsheet String(delimiter (Tab)="\r", array=w538, 3:w580) -> (spreadsheet string=→"Ozone":string)
    n164 = Array To Spreadsheet String(delimiter (Tab)="\r", array=w463, 3:w569) -> (spreadsheet string=→"Ambient Ozone":string)
    n165 = Array To Spreadsheet String(delimiter (Tab)="\r", array=w536, 3:w564) -> (spreadsheet string=→"SO2":string)
    n166 = Index Array(array=w362, index #1=5 ("index"), index #2=19 ("index")) -> (element #1=w369:string, element #2=w366:string)
    n167 = Array To Spreadsheet String(delimiter (Tab)="\r", array=w362, 3:w363) -> (spreadsheet string=→"PRTAFT_DLU":string)
    n168 = Select(t=w464, s=w467, f=w463) -> (s? t:f=w462:string[])
    n169 = Not Equal?(x=w369, y=w371) -> (x != y?=w370:bool)
    n170 = Not Equal?(x=w366, y=w371) -> (x != y?=w367:bool)
    n171 = Index Array(array=w536, index #1=6 ("index"), index #2=4 ("index"), index #3=3 ("index"), index #4=7 ("index"), index #5=8 ("index"), index #6=15 ("index"), index #7=24 ("index"), index #8=29 ("index")) -> (element #1=w453:string, element #2=w519:string, element #3=w514:string, element #4=w507:string, element #5=w483:string, element #6=w482:string, element #7=w390:string, element #8=w389:string)
    n172 = Index Array(array=w462, index #1=8 ("index"), index #2=11 ("index")) -> (element #1=w456:string, element #2=w457:string)
    n173 = case shown="False" w367 {
      tunnel: ["1" w599] -> w365
      tunnel: w366 -> [_ w599]
      frame False {
      }
      frame True {
      }
    }
    n174 = case shown="False" w370 {
      tunnel: ["XXXX" w601] -> w368
      tunnel: w369 -> [_ w601]
      frame False {
      }
      frame True {
      }
    }
    n175 = Index Array(array=w538, index #1=6 ("index"), index #2=4 ("index"), index #3=3 ("index"), index #4=7 ("index"), index #5=9 ("index"), index #6=14 ("index"), index #7=15 ("index")) -> (element #1=w532:string, element #2=w520:string, element #3=w515:string, element #4=w500:string, element #5=w473:string, element #6=w472:string, element #7=w471:string)
    n176 = Scan Value(string=w456, format string="%f") -> (value=→"2B Ozone concentration":dbl)  [unwired: 1 in, 1 out]
    n177 = Scan Value(string=w457, format string="%f") -> (value=→"2B Ozone flow rate":dbl)  [unwired: 1 in, 1 out]
    n178 = Scan Value(string=w390, format string="%f") -> (value=→"TEI43i MFC2 Cal Flow":dbl)  [unwired: 1 in, 1 out]
    n179 = Scan Value(string=w389, format string="%f") -> (value=→"TEI43i MFC3 Sample Flow":dbl)  [unwired: 1 in, 1 out]
    n180 = Scan Value(string=w483, format string="%f") -> (value=→"TEi43C Concentration":dbl)  [unwired: 1 in, 1 out]
    n181 = Scan Value(string=w482, format string="%f") -> (value=→"TEI43C Sample Flow":dbl)  [unwired: 1 in, 1 out]
    n182 = Index Array(array=w540, index #1=6 ("index"), index #2=4 ("index"), index #3=3 ("index"), index #4=7 ("index"), index #5=8 ("index"), index #6=9 ("index"), index #7=10 ("index"), index #8=17 ("index"), index #9=16 ("index"), index #10=11 ("index"), index #11=12 ("index"), index #12=21 ("index")) -> (element #1=w534:string, element #2=w522:string, element #3=w517:string, element #4=w502:string, element #5=w414:string, element #6=w411:string, element #7=w406:string, element #8=w404:string, element #9=w401:string, element #10=w396:string, element #11=w395:string, element #12=w382:string)
    n183 = local write "Flight Number"(w368) -> ()
    n184 = local write "WoW Flag"(w365) -> ()
    n185 = Index Array(array=w561, index #1=2 ("index"), index #2=27 ("index"), index #3=28 ("index"), index #4=29 ("index"), index #5=30 ("index"), index #6=31 ("index"), index #7=6 ("index"), index #8=4 ("index"), index #9=3 ("index"), index #10=8 ("index"), index #11=14 ("index"), index #12=16 ("index"), index #13=19 ("index"), index #14=12 ("index"), index #15=13 ("index"), index #16=10 ("index"), index #17=11 ("index")) -> (element #1=w424:string, element #2=w504:string, element #3=w551:string, element #4=w545:string, element #5=w543:string, element #6=w544:string, element #7=w533:string, element #8=w521:string, element #9=w516:string, element #10=w505:string, element #11=w492:string, element #12=w489:string, element #13=w488:string, element #14=w448:string, element #15=w447:string, element #16=w378:string, element #17=w357:string)
    n186 = Decimal String To Number(string=w424) -> (number=w422:i32)  [unwired: 2 in, 1 out]
    n187 = call "Find_Data_SubVI.vi"("FGGA"=w534, "CO"=w533, "Ozone"=w532, "SO2"=w453) -> ("Output Value"=→"CPU Total %":dbl)  [unwired: 11 in]
    n188 = call "Find_Data_SubVI.vi"("FGGA"=w522, "CO"=w521, "Ozone"=w520, "SO2"=w519) -> ("Output Value"=→"MFM":dbl)  [unwired: 11 in]
    n189 = call "Find_Data_SubVI.vi"("FGGA"=w517, "CO"=w516, "Ozone"=w515, "SO2"=w514) -> ("Output Value"=w513:dbl)  [unwired: 11 in]
    n190 = call "Find_Data_SubVI.vi"("FGGA"=w502, "CO"=w505, "Ozone"=w500, "SO2"=w507) -> ("Output Value"=→"USB Disk Space Used %":dbl)  [unwired: 11 in]
    n191 = Not Equal To 0?(x=w513) -> (x != 0?=→"PTP Sync":bool)
    n192 = Add(x=w422, y=u32 2082844800) -> (x+y=w421:u32)
    n193 = Scan Value(string=w382, format string="%f") -> (value=→"MFC1 Cal Flow":dbl)  [unwired: 1 in, 1 out]
    n194 = Scan Value(string=w395, format string="%f") -> (value=→"Cell temperature":dbl)  [unwired: 1 in, 1 out]
    n195 = Scan Value(string=w396, format string="%f") -> (value=→"Cell pressure":dbl)  [unwired: 1 in, 1 out]
    n196 = Scan Value(string=w401, format string="%f") -> (value=→"CH4 Dry":dbl)  [unwired: 1 in, 1 out]
    n197 = Scan Value(string=w404, format string="%f") -> (value=→"CO2 Dry":dbl)  [unwired: 1 in, 1 out]
    n198 = Scan Value(string=w406, format string="%f") -> (value=→"H2O":dbl)  [unwired: 1 in, 1 out]
    n199 = Scan Value(string=w411, format string="%f") -> (value=→"CO2":dbl)  [unwired: 1 in, 1 out]
    n200 = Scan Value(string=w414, format string="%f") -> (value=→"CH4":dbl)  [unwired: 1 in, 1 out]
    n201 = Scan Value(string=w544, format string="%f") -> (value=→"Std\nContent (barG)":dbl)  [unwired: 1 in, 1 out]
    n202 = Scan Value(string=w504, format string="%d", default (0 dbl)=u32 0) -> (value=w558:u32)  [unwired: 1 out]
    n203 = Scan Value(string=w543, format string="%f") -> (value=→"N2\nContent (barG)":dbl)  [unwired: 1 in, 1 out]
    n204 = Scan Value(string=w545, format string="%f") -> (value=→"CO2\nContent (barG)":dbl)  [unwired: 1 in, 1 out]
    n205 = Scan Value(string=w551, format string="%f") -> (value=→"CO2 Pressure\nDelivery (PSIA)":dbl)  [unwired: 1 in, 1 out]
    n206 = To Time Stamp(1:w421) -> (0:w428:timestamp)
    n207 = Scan Value(string=w492, format string="%f") -> (value=→"Lamp Flow Controller":dbl)  [unwired: 1 in, 1 out]
    n208 = Scan Value(string=w378, format string="%f") -> (value=→"CO Concentration":dbl)  [unwired: 1 in, 1 out]
    n209 = Scan Value(string=w489, format string="%f") -> (value=→"Monochromater Flow":dbl)  [unwired: 1 in, 1 out]
    n210 = Scan Value(string=w488, format string="%f") -> (value=→"Fluorsecence Cell Pressure":dbl)  [unwired: 1 in, 1 out]
    n211 = Scan Value(string=w357, format string="%f") -> (value=→"Raw Signal (Hz)":dbl)  [unwired: 1 in, 1 out]
    n212 = Not Equal To 0?(x=w558) -> (x != 0?=→"CO CAL Status":bool)
    n213 = call "ping.vi"("Host IP Address"="192.168.101.17") -> ("connected?"=w427:bool)  [unwired: 14 in]
    n214 = Scan Value(string=w473, format string="%f") -> (value=→"TEi49C Concentration":dbl)  [unwired: 1 in, 1 out]
    n215 = Scan Value(string=w472, format string="%f") -> (value=→"TEI49C Sample Flow A":dbl)  [unwired: 1 in, 1 out]
    n216 = Scan Value(string=w471, format string="%f") -> (value=→"TEI49C Sample Flow B":dbl)  [unwired: 1 in, 1 out]
    n217 = Scan Value(string=w448, format string="%f") -> (value=w439:dbl)  [unwired: 1 in, 1 out]
    n218 = Scan Value(string=w447, format string="%f") -> (value=w431:dbl)  [unwired: 1 in, 1 out]
    n219 = Not Equal?(x=w438, y=w439) -> (x != y?=w444:bool)
    n220 = Not Equal?(x=w429, y=w431) -> (x != y?=w436:bool)
    n221 = case shown="True" w444 {
      tunnel: w445 -> [w619 w628]
      tunnel: w443 -> [w620 w627]
      tunnel: [w620 w626] -> w442
      tunnel: w428 -> [_ w622]
      tunnel: w439 -> [_ w623]
      tunnel: [w619 w625] -> w441
      tunnel: [w618 w624] -> w440
      tunnel: w439 -> [_ w624]
      tunnel: w438 -> [w618 _]
      frame False {
      }
      frame True {
        n222 = Bundle(w622, w623) -> (w621:cluster{timestamp, dbl})  [unwired: 1 in]
        n223 = Replace Array Subset(array=w628, new element=w621, index=w627) -> (w625:cluster{"time stamp":timestamp, "Y":dbl}[])
        n224 = Increment(x=w627) -> (x+1=w626:i32)
      }
    }
    "CO Sensitivity" <- w441
    n225 = case shown="True" w436 {
      tunnel: w435 -> [w608 w617]
      tunnel: w434 -> [w609 w616]
      tunnel: [w609 w615] -> w432
      tunnel: w428 -> [_ w614]
      tunnel: w431 -> [_ w613]
      tunnel: [w608 w612] -> w433
      tunnel: [w607 w611] -> w430
      tunnel: w431 -> [_ w611]
      tunnel: w429 -> [w607 _]
      frame False {
      }
      frame True {
        n226 = Bundle(w614, w613) -> (w610:cluster{timestamp, dbl})  [unwired: 1 in]
        n227 = Replace Array Subset(array=w617, new element=w610, index=w616) -> (w612:cluster{"time stamp":timestamp, "Y":dbl}[])
        n228 = Increment(x=w616) -> (x+1=w615:i32)
      }
    }
    "CO Zero" <- w433
    n229 = case shown="False" w427 {
      tunnel: w426 -> [_ w606]
      tunnel: [FALSE w603] -> w425
      frame False {
      }
      frame True {
        n230 = Select(t=FALSE, s=w606, f=TRUE) -> (s? t:f=w603:bool)
      }
    }
    "Network to cRIO live status" <- w425
    n231 = Wait (ms)(milliseconds to wait=u32 1000) -> ()  [unwired: 1 out]
  }
  n232 = Obtain Queue(name (unnamed)="FGGA_Command", element data type=w55) -> (queue out=w2:refnum<queue>, error out=w1:errorcluster)  [unwired: 3 in, 1 out]
  n233 = while {
    shift-right: [w632] -> _
    shift-left: u8 1 -> [w633]
    tunnel: w2 -> [w630]
    tunnel: w1 -> [w629]
    stop <- FALSE stop-if-true
    # "FGGA pump synchronise to WoW Wait on Wheel Flag"
    n234 = Wait (ms)(milliseconds to wait=u32 1000) -> ()  [unwired: 1 out]
    n235 = case shown="True" "FGGA pump\nsync to WoW" {
      tunnel: [w636 w641] -> w632
      tunnel: w633 -> [w636 w640]
      tunnel: w630 -> [_ w639]
      tunnel: w629 -> [_ w638]
      frame False {
      }
      frame True {
        n236 = local read "WoW Flag"() -> (w637:string)
        n237 = Scan Value(string=w637, format string="%d", default (0 dbl)=u8 0) -> (value=w641:u8)  [unwired: 1 out]
        n238 = Not Equal?(x=w641, y=w640) -> (x != y?=w644:bool)
        n239 = case shown="True" w644 {
          tunnel: w641 -> [_ w647]
          tunnel: w639 -> [_ w646]
          tunnel: w638 -> [_ w645]
          frame False {
          }
          frame True {
            n240 = Equal?(x=w647, y=u8 0) -> (x = y?=w652:bool)
            n241 = case shown="True" w652 {
              selector: w652 -> [w654 w655]
              tunnel: [w654 w655] -> w648
              frame False {
              }
              frame True {
              }
            }
            n242 = local write "FGGA Pump"(w648) -> ()
            n243 = Bundle(cluster=T4 {"Message"="", "Message Data"=variant} ("Message Cluster"), "Message"="FGGA_pump", "Message Data"=w648) -> (w649:T4)
            n244 = Enqueue Element(queue=w646, element=w649, error in (no error)=w645) -> ()  [unwired: 1 in, 3 out]
          }
        }
      }
    }
  }
  n245 = while {
    tunnel: w2 -> [w657]
    tunnel: w1 -> [w656]
    tunnel: [w659] -> _
    tunnel: w13 -> [w658]
    stop <- FALSE stop-if-true
    # "FGGA UI Event Handler Loop"
    n246 = event shown="[5] \"Confirm Flight Number\": Value Change" {
      selector: _ -> [_ _ _ _ _ _ _ _ _ _ _ _ _ _ _ _ _]
      dyn-events: _ -> [_ _ _ _ _ _ _ _ _ _ _ _ _ _ _ _ _]
      timeout: _ -> [_ _ _ _ _ _ _ _ _ _ _ _ _ _ _ _ _]
      tunnel: w657 -> [w667 w671 w678 w685 w692 w699 w706 w713 w732 w841 w1014 w1081 w1148 w1205 w1292 w1360 w1367]
      tunnel: w656 -> [w666 w670 w677 w684 w691 w698 w705 w712 w731 w840 w1013 w1080 w1147 w1204 w1291 w1359 w1366]
      tunnel: [w661 w669 w676 w683 w690 w697 w704 w711 w718 w804 w1006 w1073 w1140 w1191 w1278 w1358 w1365] -> w659
      tunnel: w658 -> [_ _ _ _ _ _ _ _ _ w828 _ _ _ _ _ _ _]
      event "V1": Value Change {
        n247 = event-data() -> ("NewVal"=w664:bool)  [unwired: 1 in]
        n248 = Bundle(cluster=T4 {"Message"="", "Message Data"=variant} ("Message Cluster"), "Message"="V1", "Message Data"=w664) -> (w662:T4)
        n249 = Enqueue Element(queue=w667, element=w662, error in (no error)=w666) -> (error out=w661:errorcluster)  [unwired: 1 in, 2 out]
      }
      event "V2": Value Change {
        n250 = event-data() -> ("NewVal"=w668:bool)  [unwired: 1 in]
        n251 = Bundle(cluster=T4 {"Message"="", "Message Data"=variant} ("Message Cluster"), "Message"="V2", "Message Data"=w668) -> (w672:T4)
        n252 = Enqueue Element(queue=w671, element=w672, error in (no error)=w670) -> (error out=w669:errorcluster)  [unwired: 1 in, 2 out]
      }
      event "V3": Value Change {
        n253 = event-data() -> ("NewVal"=w675:bool)  [unwired: 1 in]
        n254 = Bundle(cluster=T4 {"Message"="", "Message Data"=variant} ("Message Cluster"), "Message"="V3", "Message Data"=w675) -> (w679:T4)
        n255 = Enqueue Element(queue=w678, element=w679, error in (no error)=w677) -> (error out=w676:errorcluster)  [unwired: 1 in, 2 out]
      }
      event "V4": Value Change {
        n256 = event-data() -> ("NewVal"=w682:bool)  [unwired: 1 in]
        n257 = Bundle(cluster=T4 {"Message"="", "Message Data"=variant} ("Message Cluster"), "Message"="V4", "Message Data"=w682) -> (w686:T4)
        n258 = Enqueue Element(queue=w685, element=w686, error in (no error)=w684) -> (error out=w683:errorcluster)  [unwired: 1 in, 2 out]
      }
      event "FGGA Pump": Value Change {
        n259 = event-data() -> ("NewVal"=w689:bool)  [unwired: 1 in]
        n260 = Bundle(cluster=T4 {"Message"="", "Message Data"=variant} ("Message Cluster"), "Message"="FGGA_pump", "Message Data"=w689) -> (w693:T4)
        n261 = Enqueue Element(queue=w692, element=w693, error in (no error)=w691) -> (error out=w690:errorcluster)  [unwired: 1 in, 2 out]
      }
      event "Confirm Flight Number": Value Change {
        n262 = event-data() -> ()  [unwired: 1 in, 6 out]
        n263 = local read "Flight Number"() -> (w696:string)
        n264 = Bundle(cluster=T4 {"Message"="", "Message Data"=variant} ("Message Cluster"), "Message"="Flight Number", "Message Data"=w696) -> (w700:T4)
        n265 = Enqueue Element(queue=w699, element=w700, error in (no error)=w698) -> (error out=w697:errorcluster)  [unwired: 1 in, 2 out]
      }
      event "FGGA Restart": Value Change {
        n266 = event-data() -> ("NewVal"=w703:bool)  [unwired: 1 in]
        n267 = Bundle(cluster=T4 {"Message"="", "Message Data"=variant} ("Message Cluster"), "Message"="FGGA_restart", "Message Data"=w703) -> (w707:T4)
        n268 = Enqueue Element(queue=w706, element=w707, error in (no error)=w705) -> (error out=w704:errorcluster)  [unwired: 1 in, 2 out]
      }
      event "cRIO File IO Stop\n(USB Flash Drive Unmount)": Value Change {
        n269 = event-data() -> ("NewVal"=w710:bool)  [unwired: 1 in]
        n270 = Bundle(cluster=T4 {"Message"="", "Message Data"=variant} ("Message Cluster"), "Message"="Stop File Write", "Message Data"=w710) -> (w714:T4)
        n271 = Enqueue Element(queue=w713, element=w714, error in (no error)=w712) -> (error out=w711:errorcluster)  [unwired: 1 in, 2 out]
      }
      event "High Cal": Value Change {
        n272 = event-data() -> ()  [unwired: 1 in, 1 out]
        n273 = flat-sequence {
          tunnel: w732 -> [w737]
          tunnel: w731 -> [w736]
          tunnel: [w735] -> w730
          tunnel: [w734] -> w729
          tunnel: w730 -> [w753]
          tunnel: w729 -> [w752]
          tunnel: [w750] -> w727
          tunnel: [w749] -> w725
          tunnel: [w758] -> w728
          tunnel: w727 -> [w758]
          tunnel: [w757] -> w726
          tunnel: w725 -> [w757]
          tunnel: w728 -> [w768]
          tunnel: w726 -> [w767]
          tunnel: [w765] -> w723
          tunnel: [w764] -> w721
          tunnel: [w774] -> w724
          tunnel: w723 -> [w774]
          tunnel: [w773] -> w722
          tunnel: w721 -> [w773]
          tunnel: w724 -> [w784]
          tunnel: w722 -> [w783]
          tunnel: [w781] -> w720
          tunnel: [w780] -> w719
          tunnel: w720 -> [w798]
          tunnel: w719 -> [w797]
          tunnel: [w795] -> w717
          tunnel: [w803] -> w718
          tunnel: w717 -> [w803]
          frame #0 {
            w733 = TRUE
            n274 = Cluster To Array(cluster=T11 {"Message"="V2", "Message 2"="V3", "Message 3"="V4"}) -> (array=w738:string[])
            n275 = for {
              tunnel: w738 -> [w745] mode=indexing
              tunnel: w737 -> [w744]
              tunnel: w736 -> [w743]
              tunnel: [w742] -> w735
              tunnel: [w741] -> w734
              tunnel: w733 -> [w740]
              n276 = Bundle(cluster=T4 {"Message"="", "Message Data"=variant} ("Message Cluster"), "Message"=w745, "Message Data"=w740) -> (w747:T4)
              n277 = Enqueue Element(queue=w744, element=w747, error in (no error)=w743) -> (queue out=w742:refnum<queue>, error out=w741:errorcluster)  [unwired: 1 in, 1 out]
            }
            n278 = local write "V2"(w733) -> ()
            n279 = local write "V4"(w733) -> ()
            n280 = local write "V3"(w733) -> ()
          }
          frame #1 {
            n281 = local read "MFC_1 User Set Value"() -> (w748:dbl)
            n282 = local write "MFC_1\nSLPM Value"(w748) -> ()
            n283 = Bundle(cluster=T4 {"Message"="", "Message Data"=variant} ("Message Cluster"), "Message"="MFC_1", "Message Data"=w748) -> (w751:T4)
            n284 = Enqueue Element(queue=w753, element=w751, error in (no error)=w752) -> (queue out=w750:refnum<queue>, error out=w749:errorcluster)  [unwired: 1 in, 1 out]
          }
          frame #2 {
            n285 = for {
              N: 45 -> [w762]
              i -> [w761]
              n286 = Subtract(x=w762, y=w761) -> (x-y=w760:i32)
              n287 = Decrement(x=w760) -> (x-1=→"High Cal\nFlush Time Remain (sec)":i32)
              n288 = Wait (ms)(milliseconds to wait=u32 1000) -> ()  [unwired: 1 out]
            }
          }
          frame #3 {
            w766 = TRUE
            n289 = Bundle(cluster=T4 {"Message"="", "Message Data"=variant} ("Message Cluster"), "Message"="V1", "Message Data"=w766) -> (w769:T4)
            n290 = local write "V1"(w766) -> ()
            n291 = Enqueue Element(queue=w768, element=w769, error in (no error)=w767) -> (queue out=w765:refnum<queue>, error out=w764:errorcluster)  [unwired: 1 in, 1 out]
          }
          frame #4 {
            n292 = for {
              N: 60 -> [w778]
              i -> [w777]
              n293 = Subtract(x=w778, y=w777) -> (x-y=w776:i32)
              n294 = Decrement(x=w776) -> (x-1=→"High Cal\nCal Time Remain (sec)":i32)
              n295 = Wait (ms)(milliseconds to wait=u32 1000) -> ()  [unwired: 1 out]
            }
          }
          frame #5 {
            w782 = FALSE
            n296 = Cluster To Array(cluster=T12 {"Message"="V2", "Message 2"="V3", "Message 3"="V4", "Message 4"="V1"}) -> (array=w785:string[])
            n297 = for {
              tunnel: w785 -> [w792] mode=indexing
              tunnel: [w791] -> w781
              tunnel: [w790] -> w780
              tunnel: w782 -> [w789]
              tunnel: w784 -> [w788]
              tunnel: w783 -> [w787]
              n298 = Bundle(cluster=T4 {"Message"="", "Message Data"=variant} ("Message Cluster"), "Message"=w792, "Message Data"=w789) -> (w794:T4)
              n299 = Enqueue Element(queue=w788, element=w794, error in (no error)=w787) -> (queue out=w791:refnum<queue>, error out=w790:errorcluster)  [unwired: 1 in, 1 out]
            }
            n300 = local write "V2"(w782) -> ()
            n301 = local write "V4"(w782) -> ()
            n302 = local write "V3"(w782) -> ()
            n303 = local write "V1"(w782) -> ()
          }
          frame #6 {
            w796 = 0.0 ("MFC_1\nSLPM Value")
            n304 = local write "MFC_1\nSLPM Value"(w796) -> ()
            n305 = Bundle(cluster=T4 {"Message"="", "Message Data"=variant} ("Message Cluster"), "Message"="MFC_1", "Message Data"=w796) -> (w800:T4)
            n306 = Enqueue Element(queue=w798, element=w800, error in (no error)=w797) -> (error out=w795:errorcluster)  [unwired: 1 in, 2 out]
          }
          frame #7 {
            n307 = local write "High Cal"(FALSE ("High Cal")) -> ()
          }
        }
      }
      event "Span Cal Synchronise with\nCO": Value Change {
        n308 = event-data() -> ()  [unwired: 1 in, 1 out]
        n309 = flat-sequence {
          tunnel: w841 -> [w847]
          tunnel: w840 -> [w846]
          tunnel: [w845] -> w839
          tunnel: [w844] -> w838
          tunnel: w839 -> [w863]
          tunnel: w838 -> [w862]
          tunnel: [w860] -> w836
          tunnel: [w859] -> w834
          tunnel: [w868] -> w837
          tunnel: w836 -> [w868]
          tunnel: [w867] -> w835
          tunnel: w834 -> [w867]
          tunnel: w837 -> [w874]
          tunnel: w835 -> [w875]
          tunnel: [w875] -> w810
          tunnel: w828 -> [w876]
          tunnel: [w876] -> w808
          tunnel: [w874] -> w806
          tunnel: w810 -> [w884]
          tunnel: [w884] -> w809
          tunnel: w808 -> [w883]
          tunnel: [w883] -> w807
          tunnel: w806 -> [w881]
          tunnel: [w881] -> w805
          tunnel: [w885] -> w827
          tunnel: w809 -> [w888]
          tunnel: [w887] -> w826
          tunnel: w807 -> [w897]
          tunnel: w805 -> [w886]
          tunnel: [w900] -> w833
          tunnel: w827 -> [w900]
          tunnel: [w899] -> w832
          tunnel: w826 -> [w899]
          tunnel: w833 -> [w910]
          tunnel: w832 -> [w909]
          tunnel: [w907] -> w831
          tunnel: [w906] -> w830
          tunnel: w831 -> [w925]
          tunnel: w830 -> [w924]
          tunnel: [w922] -> w829
          tunnel: [w921] -> w823
          tunnel: w829 -> [w931]
          tunnel: [w931] -> w825
          tunnel: [w929] -> w824
          tunnel: w823 -> [w929]
          tunnel: w825 -> [w936]
          tunnel: w824 -> [w938]
          tunnel: [w935] -> w822
          tunnel: [w932] -> w821
          tunnel: w822 -> [w952]
          tunnel: w821 -> [w950]
          tunnel: [w949] -> w820
          tunnel: [w948] -> w817
          tunnel: w820 -> [w957]
          tunnel: [w957] -> w819
          tunnel: [w956] -> w818
          tunnel: w817 -> [w956]
          tunnel: w819 -> [w969]
          tunnel: w818 -> [w967]
          tunnel: [w965] -> w815
          tunnel: [w964] -> w813
          tunnel: [w973] -> w816
          tunnel: w815 -> [w973]
          tunnel: [w972] -> w814
          tunnel: w813 -> [w972]
          tunnel: w816 -> [w984]
          tunnel: w814 -> [w983]
          tunnel: [w981] -> w812
          tunnel: [w980] -> w811
          tunnel: w812 -> [w999]
          tunnel: w811 -> [w998]
          tunnel: [w995] -> w804
          frame #0 {
            w843 = TRUE
            n310 = Cluster To Array(cluster=T11 {"Message"="V2", "Message 2"="V3", "Message 3"="V4"}) -> (array=w848:string[])
            n311 = for {
              tunnel: w848 -> [w855] mode=indexing
              tunnel: w847 -> [w854]
              tunnel: w846 -> [w853]
              tunnel: [w852] -> w845
              tunnel: [w851] -> w844
              tunnel: w843 -> [w850]
              n312 = Bundle(cluster=T4 {"Message"="", "Message Data"=variant} ("Message Cluster"), "Message"=w855, "Message Data"=w850) -> (w857:T4)
              n313 = Enqueue Element(queue=w854, element=w857, error in (no error)=w853) -> (queue out=w852:refnum<queue>, error out=w851:errorcluster)  [unwired: 1 in, 1 out]
            }
            n314 = local write "High Cal"(TRUE ("High Cal")) -> ()
            n315 = local write "V2"(w843) -> ()
            n316 = local write "V4"(w843) -> ()
            n317 = local write "V3"(w843) -> ()
          }
          frame #1 {
            n318 = local read "MFC_1 User Set Value"() -> (w858:dbl)
            n319 = local write "MFC_1\nSLPM Value"(w858) -> ()
            n320 = Bundle(cluster=T4 {"Message"="", "Message Data"=variant} ("Message Cluster"), "Message"="MFC_1", "Message Data"=w858) -> (w861:T4)
            n321 = Enqueue Element(queue=w863, element=w861, error in (no error)=w862) -> (queue out=w860:refnum<queue>, error out=w859:errorcluster)  [unwired: 1 in, 1 out]
          }
          frame #2 {
            n322 = for {
              N: 45 -> [w872]
              i -> [w871]
              n323 = Subtract(x=w872, y=w871) -> (x-y=w870:i32)
              n324 = Decrement(x=w870) -> (x-1=w869:i32)
              n325 = local write "High Cal\nFlush Time Remain (sec)"(w869) -> ()
              n326 = Wait (ms)(milliseconds to wait=u32 1000) -> ()  [unwired: 1 out]
            }
          }
          frame #3 {
            n327 = Bundle(cluster=T4 {"Message"="", "Message Data"=variant} ("Message Cluster"), "Message"="CO CAL", "Message Data"=TRUE) -> (w878:T4)
            n328 = Enqueue Element(queue=w876, element=w878) -> ()  [unwired: 2 in, 3 out]
          }
          frame #4 {
            # "To Ensure\nCO CAL\nis certain"
            n329 = Wait (ms)(milliseconds to wait=u32 1000) -> ()  [unwired: 1 out]
          }
          frame #5 {
            w892 = TRUE
            n330 = Bundle(cluster=T4 {"Message"="", "Message Data"=variant} ("Message Cluster"), "Message"="CO CAL", "Message Data"=FALSE) -> (w893:T4)
            n331 = Bundle(cluster=T4 {"Message"="", "Message Data"=variant} ("Message Cluster"), "Message"="V1", "Message Data"=w892) -> (w891:T4)
            n332 = local write "V1"(w892) -> ()
            n333 = Enqueue Element(queue=w897, element=w893) -> ()  [unwired: 2 in, 3 out]
            n334 = Enqueue Element(queue=w886, element=w891, error in (no error)=w888) -> (queue out=w885:refnum<queue>, error out=w887:errorcluster)  [unwired: 1 in, 1 out]
          }
          frame #6 {
            n335 = for {
              N: 60 -> [w904]
              i -> [w903]
              n336 = Subtract(x=w904, y=w903) -> (x-y=w902:i32)
              n337 = Decrement(x=w902) -> (x-1=w901:i32)
              n338 = local write "High Cal\nCal Time Remain (sec)"(w901) -> ()
              n339 = Wait (ms)(milliseconds to wait=u32 1000) -> ()  [unwired: 1 out]
            }
          }
          frame #7 {
            w908 = FALSE
            n340 = Cluster To Array(cluster=T12 {"Message"="V2", "Message 2"="V3", "Message 3"="V4", "Message 4"="V1"}) -> (array=w911:string[])
            n341 = for {
              tunnel: w911 -> [w918] mode=indexing
              tunnel: [w917] -> w907
              tunnel: [w916] -> w906
              tunnel: w908 -> [w915]
              tunnel: w910 -> [w914]
              tunnel: w909 -> [w913]
              n342 = Bundle(cluster=T4 {"Message"="", "Message Data"=variant} ("Message Cluster"), "Message"=w918, "Message Data"=w915) -> (w920:T4)
              n343 = Enqueue Element(queue=w914, element=w920, error in (no error)=w913) -> (queue out=w917:refnum<queue>, error out=w916:errorcluster)  [unwired: 1 in, 1 out]
            }
            n344 = local write "V2"(w908) -> ()
            n345 = local write "V4"(w908) -> ()
            n346 = local write "V3"(w908) -> ()
            n347 = local write "V1"(w908) -> ()
          }
          frame #8 {
            w923 = 0.0 ("MFC_1\nSLPM Value")
            n348 = local write "MFC_1\nSLPM Value"(w923) -> ()
            n349 = Bundle(cluster=T4 {"Message"="", "Message Data"=variant} ("Message Cluster"), "Message"="MFC_1", "Message Data"=w923) -> (w927:T4)
            n350 = Enqueue Element(queue=w925, element=w927, error in (no error)=w924) -> (queue out=w921:refnum<queue>, error out=w922:errorcluster)  [unwired: 1 in, 1 out]
          }
          frame #9 {
            n351 = local write "High Cal"(FALSE ("High Cal")) -> ()
          }
          frame #10 {
            w933 = TRUE
            n352 = Cluster To Array(cluster=cluster{"Message":string, "Message 3":string} {"Message"="V2", "Message 3"="V4"}) -> (array=w939:string[])
            n353 = for {
              tunnel: w939 -> [w945] mode=indexing
              tunnel: w938 -> [w944]
              tunnel: [w943] -> w932
              tunnel: [w942] -> w935
              tunnel: w933 -> [w941]
              tunnel: w936 -> [w940]
              n354 = Bundle(cluster=T4 {"Message"="", "Message Data"=variant} ("Message Cluster"), "Message"=w945, "Message Data"=w941) -> (w947:T4)
              n355 = Enqueue Element(queue=w944, element=w947, error in (no error)=w940) -> (queue out=w943:refnum<queue>, error out=w942:errorcluster)  [unwired: 1 in, 1 out]
            }
            n356 = local write "V4"(w933) -> ()
            n357 = local write "V2"(w933) -> ()
            n358 = local write "Low Cal"(TRUE ("Low Cal")) -> ()
          }
          frame #11 {
            n359 = local read "MFC_1 User Set Value"() -> (w953:dbl)
            n360 = local write "MFC_1\nSLPM Value"(w953) -> ()
            n361 = Bundle(cluster=T4 {"Message"="", "Message Data"=variant} ("Message Cluster"), "Message"="MFC_1", "Message Data"=w953) -> (w954:T4)
            n362 = Enqueue Element(queue=w950, element=w954, error in (no error)=w952) -> (queue out=w949:refnum<queue>, error out=w948:errorcluster)  [unwired: 1 in, 1 out]
          }
          frame #12 {
            n363 = for {
              N: 45 -> [w962]
              i -> [w961]
              n364 = Subtract(x=w962, y=w961) -> (x-y=w960:i32)
              n365 = Decrement(x=w960) -> (x-1=w959:i32)
              n366 = local write "Low Cal\nFlush Time Remain (sec)"(w959) -> ()
              n367 = Wait (ms)(milliseconds to wait=u32 1000) -> ()  [unwired: 1 out]
            }
          }
          frame #13 {
            w966 = TRUE
            n368 = local write "V1"(w966) -> ()
            n369 = Bundle(cluster=T4 {"Message"="", "Message Data"=variant} ("Message Cluster"), "Message"="V1", "Message Data"=w966) -> (w970:T4)
            n370 = Enqueue Element(queue=w969, element=w970, error in (no error)=w967) -> (queue out=w965:refnum<queue>, error out=w964:errorcluster)  [unwired: 1 in, 1 out]
          }
          frame #14 {
            n371 = for {
              N: 60 -> [w978]
              i -> [w977]
              n372 = Subtract(x=w978, y=w977) -> (x-y=w976:i32)
              n373 = Decrement(x=w976) -> (x-1=w975:i32)
              n374 = local write "Low Cal\nCal Time Remain (sec)"(w975) -> ()
              n375 = Wait (ms)(milliseconds to wait=u32 1000) -> ()  [unwired: 1 out]
            }
          }
          frame #15 {
            w982 = FALSE
            n376 = Cluster To Array(cluster=T13 {"Message"="V2", "Message 3"="V4", "Message 4"="V1"}) -> (array=w985:string[])
            n377 = for {
              tunnel: w985 -> [w992] mode=indexing
              tunnel: [w991] -> w981
              tunnel: [w990] -> w980
              tunnel: w982 -> [w989]
              tunnel: w984 -> [w988]
              tunnel: w983 -> [w987]
              n378 = Bundle(cluster=T4 {"Message"="", "Message Data"=variant} ("Message Cluster"), "Message"=w992, "Message Data"=w989) -> (w994:T4)
              n379 = Enqueue Element(queue=w988, element=w994, error in (no error)=w987) -> (queue out=w991:refnum<queue>, error out=w990:errorcluster)  [unwired: 1 in, 1 out]
            }
            n380 = local write "V1"(w982) -> ()
            n381 = local write "V2"(w982) -> ()
            n382 = local write "V4"(w982) -> ()
          }
          frame #16 {
            w996 = FALSE
            w997 = 0.0 ("MFC_1\nSLPM Value")
            n383 = local write "Span Cal Synchronise with\nCO"(w996) -> ()
            n384 = local write "MFC_1\nSLPM Value"(w997) -> ()
            n385 = local write "Low Cal"(w996) -> ()
            n386 = Bundle(cluster=T4 {"Message"="", "Message Data"=variant} ("Message Cluster"), "Message"="MFC_1", "Message Data"=w997) -> (w1001:T4)
            n387 = Enqueue Element(queue=w999, element=w1001, error in (no error)=w998) -> (error out=w995:errorcluster)  [unwired: 1 in, 2 out]
          }
        }
      }
      event "Flush High Tank": Value Change {
        n388 = event-data() -> ()  [unwired: 1 in, 1 out]
        n389 = flat-sequence {
          tunnel: w1014 -> [w1019]
          tunnel: w1013 -> [w1018]
          tunnel: [w1017] -> w1012
          tunnel: [w1016] -> w1011
          tunnel: w1012 -> [w1035]
          tunnel: w1011 -> [w1034]
          tunnel: [w1032] -> w1010
          tunnel: [w1031] -> w1009
          tunnel: w1010 -> [w1038]
          tunnel: w1009 -> [w1039]
          tunnel: [w1039] -> w1004
          tunnel: [w1038] -> w1003
          tunnel: [w1049] -> w1008
          tunnel: [w1048] -> w1007
          tunnel: w1004 -> [w1047]
          tunnel: w1003 -> [w1046]
          tunnel: w1008 -> [w1064]
          tunnel: w1007 -> [w1063]
          tunnel: [w1061] -> w1005
          tunnel: [w1069] -> w1006
          tunnel: w1005 -> [w1069]
          frame #0 {
            w1015 = TRUE
            n390 = Cluster To Array(cluster=T11 {"Message"="V2", "Message 2"="V3", "Message 3"="V4"}) -> (array=w1020:string[])
            n391 = for {
              tunnel: w1020 -> [w1027] mode=indexing
              tunnel: w1019 -> [w1026]
              tunnel: w1018 -> [w1025]
              tunnel: [w1024] -> w1017
              tunnel: [w1023] -> w1016
              tunnel: w1015 -> [w1022]
              n392 = Bundle(cluster=T4 {"Message"="", "Message Data"=variant} ("Message Cluster"), "Message"=w1027, "Message Data"=w1022) -> (w1029:T4)
              n393 = Enqueue Element(queue=w1026, element=w1029, error in (no error)=w1025) -> (queue out=w1024:refnum<queue>, error out=w1023:errorcluster)  [unwired: 1 in, 1 out]
            }
            n394 = local write "V2"(w1015) -> ()
            n395 = local write "V4"(w1015) -> ()
            n396 = local write "V3"(w1015) -> ()
          }
          frame #1 {
            n397 = local read "MFC_1 User Set Value"() -> (w1030:dbl)
            n398 = local write "MFC_1\nSLPM Value"(w1030) -> ()
            n399 = Bundle(cluster=T4 {"Message"="", "Message Data"=variant} ("Message Cluster"), "Message"="MFC_1", "Message Data"=w1030) -> (w1033:T4)
            n400 = Enqueue Element(queue=w1035, element=w1033, error in (no error)=w1034) -> (queue out=w1032:refnum<queue>, error out=w1031:errorcluster)  [unwired: 1 in, 1 out]
          }
          frame #2 {
            n401 = for {
              N: 15 -> [w1044]
              i -> [w1043]
              n402 = Subtract(x=w1044, y=w1043) -> (x-y=w1042:i32)
              n403 = Decrement(x=w1042) -> (x-1=→"Flush High Tank\nTime Remain (sec)":i32)
              n404 = Wait (ms)(milliseconds to wait=u32 1000) -> ()  [unwired: 1 out]
            }
          }
          frame #3 {
            w1050 = FALSE
            n405 = Cluster To Array(cluster=T11 {"Message"="V2", "Message 2"="V3", "Message 3"="V4"}) -> (array=w1051:string[])
            n406 = for {
              tunnel: w1051 -> [w1058] mode=indexing
              tunnel: [w1057] -> w1049
              tunnel: [w1056] -> w1048
              tunnel: w1050 -> [w1055]
              tunnel: w1046 -> [w1054]
              tunnel: w1047 -> [w1053]
              n407 = Bundle(cluster=T4 {"Message"="", "Message Data"=variant} ("Message Cluster"), "Message"=w1058, "Message Data"=w1055) -> (w1060:T4)
              n408 = Enqueue Element(queue=w1054, element=w1060, error in (no error)=w1053) -> (queue out=w1057:refnum<queue>, error out=w1056:errorcluster)  [unwired: 1 in, 1 out]
            }
            n409 = local write "V2"(w1050) -> ()
            n410 = local write "V4"(w1050) -> ()
            n411 = local write "V3"(w1050) -> ()
          }
          frame #4 {
            w1062 = 0.0 ("MFC_1\nSLPM Value")
            n412 = local write "MFC_1\nSLPM Value"(w1062) -> ()
            n413 = Bundle(cluster=T4 {"Message"="", "Message Data"=variant} ("Message Cluster"), "Message"="MFC_1", "Message Data"=w1062) -> (w1066:T4)
            n414 = Enqueue Element(queue=w1064, element=w1066, error in (no error)=w1063) -> (error out=w1061:errorcluster)  [unwired: 1 in, 2 out]
          }
          frame #5 {
            n415 = local write "Flush High Tank"(FALSE ("High Cal")) -> ()
          }
        }
      }
      event "Flush Low Tank": Value Change {
        n416 = event-data() -> ()  [unwired: 1 in, 1 out]
        n417 = flat-sequence {
          tunnel: w1081 -> [w1086]
          tunnel: w1080 -> [w1085]
          tunnel: [w1084] -> w1079
          tunnel: [w1083] -> w1078
          tunnel: w1079 -> [w1102]
          tunnel: w1078 -> [w1101]
          tunnel: [w1099] -> w1077
          tunnel: [w1098] -> w1076
          tunnel: w1077 -> [w1105]
          tunnel: w1076 -> [w1106]
          tunnel: [w1106] -> w1071
          tunnel: [w1105] -> w1070
          tunnel: [w1116] -> w1075
          tunnel: [w1115] -> w1074
          tunnel: w1071 -> [w1114]
          tunnel: w1070 -> [w1113]
          tunnel: w1075 -> [w1131]
          tunnel: w1074 -> [w1130]
          tunnel: [w1128] -> w1072
          tunnel: [w1136] -> w1073
          tunnel: w1072 -> [w1136]
          frame #0 {
            w1082 = TRUE
            n418 = Cluster To Array(cluster=cluster{"Message":string, "Message 3":string} {"Message"="V2", "Message 3"="V4"}) -> (array=w1087:string[])
            n419 = for {
              tunnel: w1087 -> [w1094] mode=indexing
              tunnel: w1086 -> [w1093]
              tunnel: w1085 -> [w1092]
              tunnel: [w1091] -> w1084
              tunnel: [w1090] -> w1083
              tunnel: w1082 -> [w1089]
              n420 = Bundle(cluster=T4 {"Message"="", "Message Data"=variant} ("Message Cluster"), "Message"=w1094, "Message Data"=w1089) -> (w1096:T4)
              n421 = Enqueue Element(queue=w1093, element=w1096, error in (no error)=w1092) -> (queue out=w1091:refnum<queue>, error out=w1090:errorcluster)  [unwired: 1 in, 1 out]
            }
            n422 = local write "V2"(w1082) -> ()
            n423 = local write "V4"(w1082) -> ()
          }
          frame #1 {
            n424 = local read "MFC_1 User Set Value"() -> (w1097:dbl)
            n425 = local write "MFC_1\nSLPM Value"(w1097) -> ()
            n426 = Bundle(cluster=T4 {"Message"="", "Message Data"=variant} ("Message Cluster"), "Message"="MFC_1", "Message Data"=w1097) -> (w1100:T4)
            n427 = Enqueue Element(queue=w1102, element=w1100, error in (no error)=w1101) -> (queue out=w1099:refnum<queue>, error out=w1098:errorcluster)  [unwired: 1 in, 1 out]
          }
          frame #2 {
            n428 = for {
              N: 15 -> [w1111]
              i -> [w1110]
              n429 = Subtract(x=w1111, y=w1110) -> (x-y=w1109:i32)
              n430 = Decrement(x=w1109) -> (x-1=→"Flush Low Tank\nTime Remain (sec)":i32)
              n431 = Wait (ms)(milliseconds to wait=u32 1000) -> ()  [unwired: 1 out]
            }
          }
          frame #3 {
            w1117 = FALSE
            n432 = Cluster To Array(cluster=cluster{"Message":string, "Message 3":string} {"Message"="V2", "Message 3"="V4"}) -> (array=w1118:string[])
            n433 = for {
              tunnel: w1118 -> [w1125] mode=indexing
              tunnel: [w1124] -> w1116
              tunnel: [w1123] -> w1115
              tunnel: w1117 -> [w1122]
              tunnel: w1113 -> [w1121]
              tunnel: w1114 -> [w1120]
              n434 = Bundle(cluster=T4 {"Message"="", "Message Data"=variant} ("Message Cluster"), "Message"=w1125, "Message Data"=w1122) -> (w1127:T4)
              n435 = Enqueue Element(queue=w1121, element=w1127, error in (no error)=w1120) -> (queue out=w1124:refnum<queue>, error out=w1123:errorcluster)  [unwired: 1 in, 1 out]
            }
            n436 = local write "V2"(w1117) -> ()
            n437 = local write "V4"(w1117) -> ()
          }
          frame #4 {
            w1129 = 0.0 ("MFC_1\nSLPM Value")
            n438 = local write "MFC_1\nSLPM Value"(w1129) -> ()
            n439 = Bundle(cluster=T4 {"Message"="", "Message Data"=variant} ("Message Cluster"), "Message"="MFC_1", "Message Data"=w1129) -> (w1133:T4)
            n440 = Enqueue Element(queue=w1131, element=w1133, error in (no error)=w1130) -> (error out=w1128:errorcluster)  [unwired: 1 in, 2 out]
          }
          frame #5 {
            n441 = local write "Flush Low Tank"(FALSE ("High Cal")) -> ()
          }
        }
      }
      event "Flush Target Tank": Value Change {
        n442 = event-data() -> ()  [unwired: 1 in, 1 out]
        n443 = flat-sequence {
          tunnel: w1148 -> [w1156]
          tunnel: w1147 -> [w1155]
          tunnel: [w1154] -> w1146
          tunnel: [w1153] -> w1145
          tunnel: w1146 -> [w1162]
          tunnel: w1145 -> [w1161]
          tunnel: [w1159] -> w1144
          tunnel: [w1158] -> w1143
          tunnel: w1144 -> [w1165]
          tunnel: w1143 -> [w1166]
          tunnel: [w1166] -> w1138
          tunnel: [w1165] -> w1137
          tunnel: [w1179] -> w1142
          tunnel: [w1178] -> w1141
          tunnel: w1138 -> [w1177]
          tunnel: w1137 -> [w1176]
          tunnel: w1142 -> [w1184]
          tunnel: w1141 -> [w1183]
          tunnel: [w1181] -> w1139
          tunnel: [w1189] -> w1140
          tunnel: w1139 -> [w1189]
          frame #0 {
            w1152 = TRUE
            n444 = local write "V4"(w1152) -> ()
            n445 = Bundle(cluster=T4 {"Message"="", "Message Data"=variant} ("Message Cluster"), "Message"="V4" ("Message 3"), "Message Data"=w1152) -> (w1151:T4)
            n446 = Enqueue Element(queue=w1156, element=w1151, error in (no error)=w1155) -> (queue out=w1154:refnum<queue>, error out=w1153:errorcluster)  [unwired: 1 in, 1 out]
          }
          frame #1 {
            n447 = local read "MFC_1 User Set Value"() -> (w1157:dbl)
            n448 = local write "MFC_1\nSLPM Value"(w1157) -> ()
            n449 = Bundle(cluster=T4 {"Message"="", "Message Data"=variant} ("Message Cluster"), "Message"="MFC_1", "Message Data"=w1157) -> (w1160:T4)
            n450 = Enqueue Element(queue=w1162, element=w1160, error in (no error)=w1161) -> (queue out=w1159:refnum<queue>, error out=w1158:errorcluster)  [unwired: 1 in, 1 out]
          }
          frame #2 {
            n451 = for {
              N: 15 -> [w1171]
              i -> [w1170]
              n452 = Subtract(x=w1171, y=w1170) -> (x-y=w1169:i32)
              n453 = Decrement(x=w1169) -> (x-1=→"Flush Target Tank\nTime Remain (sec)":i32)
              n454 = Wait (ms)(milliseconds to wait=u32 1000) -> ()  [unwired: 1 out]
            }
          }
          frame #3 {
            w1180 = FALSE
            n455 = Bundle(cluster=T4 {"Message"="", "Message Data"=variant} ("Message Cluster"), "Message"="V4" ("Message 3"), "Message Data"=w1180) -> (w1175:T4)
            n456 = local write "V4"(w1180) -> ()
            n457 = Enqueue Element(queue=w1176, element=w1175, error in (no error)=w1177) -> (queue out=w1179:refnum<queue>, error out=w1178:errorcluster)  [unwired: 1 in, 1 out]
          }
          frame #4 {
            w1182 = 0.0 ("MFC_1\nSLPM Value")
            n458 = local write "MFC_1\nSLPM Value"(w1182) -> ()
            n459 = Bundle(cluster=T4 {"Message"="", "Message Data"=variant} ("Message Cluster"), "Message"="MFC_1", "Message Data"=w1182) -> (w1186:T4)
            n460 = Enqueue Element(queue=w1184, element=w1186, error in (no error)=w1183) -> (error out=w1181:errorcluster)  [unwired: 1 in, 2 out]
          }
          frame #5 {
            n461 = local write "Flush Target Tank"(FALSE ("High Cal")) -> ()
          }
        }
      }
      event "Low Cal": Value Change {
        n462 = event-data() -> ()  [unwired: 1 in, 1 out]
        n463 = flat-sequence {
          tunnel: w1205 -> [w1210]
          tunnel: w1204 -> [w1209]
          tunnel: [w1208] -> w1203
          tunnel: [w1207] -> w1202
          tunnel: w1203 -> [w1226]
          tunnel: w1202 -> [w1225]
          tunnel: [w1223] -> w1200
          tunnel: [w1222] -> w1198
          tunnel: [w1231] -> w1201
          tunnel: w1200 -> [w1231]
          tunnel: [w1230] -> w1199
          tunnel: w1198 -> [w1230]
          tunnel: w1201 -> [w1241]
          tunnel: w1199 -> [w1240]
          tunnel: [w1238] -> w1196
          tunnel: [w1237] -> w1194
          tunnel: [w1247] -> w1197
          tunnel: w1196 -> [w1247]
          tunnel: [w1246] -> w1195
          tunnel: w1194 -> [w1246]
          tunnel: w1197 -> [w1257]
          tunnel: w1195 -> [w1256]
          tunnel: [w1254] -> w1193
          tunnel: [w1253] -> w1192
          tunnel: w1193 -> [w1271]
          tunnel: w1192 -> [w1270]
          tunnel: [w1268] -> w1190
          tunnel: [w1276] -> w1191
          tunnel: w1190 -> [w1276]
          frame #0 {
            w1206 = TRUE
            n464 = Cluster To Array(cluster=cluster{"Message":string, "Message 3":string} {"Message"="V2", "Message 3"="V4"}) -> (array=w1211:string[])
            n465 = for {
              tunnel: w1211 -> [w1218] mode=indexing
              tunnel: w1210 -> [w1217]
              tunnel: w1209 -> [w1216]
              tunnel: [w1215] -> w1208
              tunnel: [w1214] -> w1207
              tunnel: w1206 -> [w1213]
              n466 = Bundle(cluster=T4 {"Message"="", "Message Data"=variant} ("Message Cluster"), "Message"=w1218, "Message Data"=w1213) -> (w1220:T4)
              n467 = Enqueue Element(queue=w1217, element=w1220, error in (no error)=w1216) -> (queue out=w1215:refnum<queue>, error out=w1214:errorcluster)  [unwired: 1 in, 1 out]
            }
            n468 = local write "V2"(w1206) -> ()
            n469 = local write "V4"(w1206) -> ()
          }
          frame #1 {
            n470 = local read "MFC_1 User Set Value"() -> (w1221:dbl)
            n471 = local write "MFC_1\nSLPM Value"(w1221) -> ()
            n472 = Bundle(cluster=T4 {"Message"="", "Message Data"=variant} ("Message Cluster"), "Message"="MFC_1", "Message Data"=w1221) -> (w1224:T4)
            n473 = Enqueue Element(queue=w1226, element=w1224, error in (no error)=w1225) -> (queue out=w1223:refnum<queue>, error out=w1222:errorcluster)  [unwired: 1 in, 1 out]
          }
          frame #2 {
            n474 = for {
              N: 45 -> [w1235]
              i -> [w1234]
              n475 = Subtract(x=w1235, y=w1234) -> (x-y=w1233:i32)
              n476 = Decrement(x=w1233) -> (x-1=→"Low Cal\nFlush Time Remain (sec)":i32)
              n477 = Wait (ms)(milliseconds to wait=u32 1000) -> ()  [unwired: 1 out]
            }
          }
          frame #3 {
            w1239 = TRUE
            n478 = Bundle(cluster=T4 {"Message"="", "Message Data"=variant} ("Message Cluster"), "Message"="V1", "Message Data"=w1239) -> (w1242:T4)
            n479 = local write "V1"(w1239) -> ()
            n480 = Enqueue Element(queue=w1241, element=w1242, error in (no error)=w1240) -> (queue out=w1238:refnum<queue>, error out=w1237:errorcluster)  [unwired: 1 in, 1 out]
          }
          frame #4 {
            n481 = for {
              N: 60 -> [w1251]
              i -> [w1250]
              n482 = Subtract(x=w1251, y=w1250) -> (x-y=w1249:i32)
              n483 = Decrement(x=w1249) -> (x-1=→"Low Cal\nCal Time Remain (sec)":i32)
              n484 = Wait (ms)(milliseconds to wait=u32 1000) -> ()  [unwired: 1 out]
            }
          }
          frame #5 {
            w1255 = FALSE
            n485 = Cluster To Array(cluster=T13 {"Message"="V2", "Message 3"="V4", "Message 4"="V1"}) -> (array=w1258:string[])
            n486 = for {
              tunnel: w1258 -> [w1265] mode=indexing
              tunnel: [w1264] -> w1254
              tunnel: [w1263] -> w1253
              tunnel: w1255 -> [w1262]
              tunnel: w1257 -> [w1261]
              tunnel: w1256 -> [w1260]
              n487 = Bundle(cluster=T4 {"Message"="", "Message Data"=variant} ("Message Cluster"), "Message"=w1265, "Message Data"=w1262) -> (w1267:T4)
              n488 = Enqueue Element(queue=w1261, element=w1267, error in (no error)=w1260) -> (queue out=w1264:refnum<queue>, error out=w1263:errorcluster)  [unwired: 1 in, 1 out]
            }
            n489 = local write "V2"(w1255) -> ()
            n490 = local write "V4"(w1255) -> ()
            n491 = local write "V1"(w1255) -> ()
          }
          frame #6 {
            w1269 = 0.0 ("MFC_1\nSLPM Value")
            n492 = local write "MFC_1\nSLPM Value"(w1269) -> ()
            n493 = Bundle(cluster=T4 {"Message"="", "Message Data"=variant} ("Message Cluster"), "Message"="MFC_1", "Message Data"=w1269) -> (w1273:T4)
            n494 = Enqueue Element(queue=w1271, element=w1273, error in (no error)=w1270) -> (error out=w1268:errorcluster)  [unwired: 1 in, 2 out]
          }
          frame #7 {
            n495 = local write "Low Cal"(FALSE ("High Cal")) -> ()
          }
        }
      }
      event "Target Cal": Value Change {
        n496 = event-data() -> ()  [unwired: 1 in, 1 out]
        n497 = flat-sequence {
          tunnel: w1292 -> [w1300]
          tunnel: w1291 -> [w1299]
          tunnel: [w1298] -> w1290
          tunnel: [w1297] -> w1289
          tunnel: w1290 -> [w1306]
          tunnel: w1289 -> [w1305]
          tunnel: [w1303] -> w1287
          tunnel: [w1302] -> w1285
          tunnel: [w1311] -> w1288
          tunnel: w1287 -> [w1311]
          tunnel: [w1310] -> w1286
          tunnel: w1285 -> [w1310]
          tunnel: w1288 -> [w1321]
          tunnel: w1286 -> [w1320]
          tunnel: [w1318] -> w1283
          tunnel: [w1317] -> w1281
          tunnel: [w1327] -> w1284
          tunnel: w1283 -> [w1327]
          tunnel: [w1326] -> w1282
          tunnel: w1281 -> [w1326]
          tunnel: w1284 -> [w1336]
          tunnel: w1282 -> [w1335]
          tunnel: [w1333] -> w1280
          tunnel: [w1334] -> w1279
          tunnel: w1280 -> [w1351]
          tunnel: w1279 -> [w1350]
          tunnel: [w1348] -> w1277
          tunnel: [w1356] -> w1278
          tunnel: w1277 -> [w1356]
          frame #0 {
            w1296 = TRUE
            n498 = local write "V4"(w1296) -> ()
            n499 = Bundle(cluster=T4 {"Message"="", "Message Data"=variant} ("Message Cluster"), "Message"="V4" ("Message 3"), "Message Data"=w1296) -> (w1295:T4)
            n500 = Enqueue Element(queue=w1300, element=w1295, error in (no error)=w1299) -> (queue out=w1298:refnum<queue>, error out=w1297:errorcluster)  [unwired: 1 in, 1 out]
          }
          frame #1 {
            n501 = local read "MFC_1 User Set Value"() -> (w1301:dbl)
            n502 = local write "MFC_1\nSLPM Value"(w1301) -> ()
            n503 = Bundle(cluster=T4 {"Message"="", "Message Data"=variant} ("Message Cluster"), "Message"="MFC_1", "Message Data"=w1301) -> (w1304:T4)
            n504 = Enqueue Element(queue=w1306, element=w1304, error in (no error)=w1305) -> (queue out=w1303:refnum<queue>, error out=w1302:errorcluster)  [unwired: 1 in, 1 out]
          }
          frame #2 {
            n505 = for {
              N: 45 -> [w1315]
              i -> [w1314]
              n506 = Subtract(x=w1315, y=w1314) -> (x-y=w1313:i32)
              n507 = Decrement(x=w1313) -> (x-1=→"Target Cal\nFlush Time Remain (sec)":i32)
              n508 = Wait (ms)(milliseconds to wait=u32 1000) -> ()  [unwired: 1 out]
            }
          }
          frame #3 {
            w1319 = TRUE
            n509 = Bundle(cluster=T4 {"Message"="", "Message Data"=variant} ("Message Cluster"), "Message"="V1", "Message Data"=w1319) -> (w1322:T4)
            n510 = local write "V1"(w1319) -> ()
            n511 = Enqueue Element(queue=w1321, element=w1322, error in (no error)=w1320) -> (queue out=w1318:refnum<queue>, error out=w1317:errorcluster)  [unwired: 1 in, 1 out]
          }
          frame #4 {
            n512 = for {
              N: 60 -> [w1331]
              i -> [w1330]
              n513 = Subtract(x=w1331, y=w1330) -> (x-y=w1329:i32)
              n514 = Decrement(x=w1329) -> (x-1=→"Target Cal\nCal Time Remain (sec)":i32)
              n515 = Wait (ms)(milliseconds to wait=u32 1000) -> ()  [unwired: 1 out]
            }
          }
          frame #5 {
            w1339 = FALSE
            n516 = Cluster To Array(cluster=cluster{"Message 3":string, "Message":string} {"Message 3"="V4", "Message"="V1"}) -> (array=w1337:string[])
            n517 = for {
              tunnel: w1337 -> [w1345] mode=indexing
              tunnel: [w1344] -> w1333
              tunnel: [w1343] -> w1334
              tunnel: w1339 -> [w1342]
              tunnel: w1336 -> [w1341]
              tunnel: w1335 -> [w1340]
              n518 = Bundle(cluster=T4 {"Message"="", "Message Data"=variant} ("Message Cluster"), "Message"=w1345, "Message Data"=w1342) -> (w1347:T4)
              n519 = Enqueue Element(queue=w1341, element=w1347, error in (no error)=w1340) -> (queue out=w1344:refnum<queue>, error out=w1343:errorcluster)  [unwired: 1 in, 1 out]
            }
            n520 = local write "V4"(w1339) -> ()
            n521 = local write "V1"(w1339) -> ()
          }
          frame #6 {
            w1349 = 0.0 ("MFC_1\nSLPM Value")
            n522 = local write "MFC_1\nSLPM Value"(w1349) -> ()
            n523 = Bundle(cluster=T4 {"Message"="", "Message Data"=variant} ("Message Cluster"), "Message"="MFC_1", "Message Data"=w1349) -> (w1353:T4)
            n524 = Enqueue Element(queue=w1351, element=w1353, error in (no error)=w1350) -> (error out=w1348:errorcluster)  [unwired: 1 in, 2 out]
          }
          frame #7 {
            n525 = local write "Target Cal"(FALSE ("High Cal")) -> ()
          }
        }
      }
      event "MFC_1\nSLPM Value": Value Change {
        n526 = event-data() -> ()  [unwired: 1 in, 1 out]
        n527 = local read "MFC_1\nSLPM Value"() -> (w1357:dbl)
        n528 = Bundle(cluster=T4 {"Message"="", "Message Data"=variant} ("Message Cluster"), "Message"="MFC_1", "Message Data"=w1357) -> (w1361:T4)
        n529 = Enqueue Element(queue=w1360, element=w1361, error in (no error)=w1359) -> (error out=w1358:errorcluster)  [unwired: 1 in, 2 out]
      }
      event "FGGA UDP Time Offset": Value Change {
        n530 = event-data() -> ("NewVal"=w1364:i32)  [unwired: 1 in, 5 out]
        n531 = Bundle(cluster=T4 {"Message"="", "Message Data"=variant} ("Message Cluster"), "Message"="UDP Time Offset", "Message Data"=w1364) -> (w1368:T4)
        n532 = Enqueue Element(queue=w1367, element=w1368, error in (no error)=w1366) -> (error out=w1365:errorcluster)  [unwired: 1 in, 2 out]
      }
    }
    "FGGA Event Error out" <- w659
  }
  n533 = Create Network Stream Writer Endpoint(6:w53, 7:10 ("writer buffer size"), 9:w55, 10:"//192.168.101.17/command/reader/FGGA" ("reader url"), 11:"/command/writer/FGGA" ("writer name")) -> (0:w52:errorcluster, 3:w51:refnum<k21>)  [unwired: 2 in]
  n534 = node-c288(w11) -> ()  [unwired: 1 out]
  n535 = while {
    tunnel: w2 -> [w1378]
    shift-right: [w1373] -> _
    shift-left: w51 -> [w1375]
    shift-right: [w1371] -> w48
    shift-left: w52 -> [w1377]
    tunnel: w1 -> [w1372]
    stop <- w1371 stop-if-true
    # "FGGA UI Command Sender"
    n536 = Dequeue Element(queue=w1378, error in (no error)=w1372) -> (element=w1374:T4)  [unwired: 1 in, 3 out]
    n537 = Unbundle By Name(w1374) -> ("Message"=w1376:string)
    n538 = case shown="\"UDP Time Offset\"" w1376 {
      tunnel: w1377 -> [w1379 w1383 w1390 w1397 w1404 w1411 w1418 w1425 w1432 w1439 w1446]
      tunnel: w1375 -> [w1380 w1386 w1393 w1400 w1407 w1414 w1421 w1428 w1435 w1442 w1449]
      tunnel: w1374 -> [_ w1385 w1392 w1399 w1406 w1413 w1420 w1427 w1434 w1441 w1448]
      tunnel: [w1379 w1382 w1389 w1396 w1403 w1410 w1417 w1424 w1431 w1438 w1445] -> w1371
      tunnel: [w1380 w1381 w1388 w1395 w1402 w1409 w1416 w1423 w1430 w1437 w1444] -> w1373
      frame "False", Default {
      }
      frame "V1" {
        n539 = shared-variable-write(w1386, w1383, w1385) -> (w1384:refnum<k21>, w1387:errorcluster)  [unwired: 1 in, 1 out]
        n540 = Flush Stream(8:w1387, 11:w1384) -> (0:w1382:errorcluster, 3:w1381:refnum<k21>)  [unwired: 2 in, 1 out]
      }
      frame "MFC_1" {
        n541 = shared-variable-write(w1393, w1390, w1392) -> (w1391:refnum<k21>, w1394:errorcluster)  [unwired: 1 in, 1 out]
        n542 = Flush Stream(8:w1394, 11:w1391) -> (0:w1389:errorcluster, 3:w1388:refnum<k21>)  [unwired: 2 in, 1 out]
      }
      frame "UDP Time Offset" {
        n543 = shared-variable-write(w1400, w1397, w1399) -> (w1398:refnum<k21>, w1401:errorcluster)  [unwired: 1 in, 1 out]
        n544 = Flush Stream(8:w1401, 11:w1398) -> (0:w1396:errorcluster, 3:w1395:refnum<k21>)  [unwired: 2 in, 1 out]
      }
      frame "V2" {
        n545 = shared-variable-write(w1407, w1404, w1406) -> (w1405:refnum<k21>, w1408:errorcluster)  [unwired: 1 in, 1 out]
        n546 = Flush Stream(8:w1408, 11:w1405) -> (0:w1403:errorcluster, 3:w1402:refnum<k21>)  [unwired: 2 in, 1 out]
      }
      frame "V3" {
        n547 = shared-variable-write(w1414, w1411, w1413) -> (w1412:refnum<k21>, w1415:errorcluster)  [unwired: 1 in, 1 out]
        n548 = Flush Stream(8:w1415, 11:w1412) -> (0:w1410:errorcluster, 3:w1409:refnum<k21>)  [unwired: 2 in, 1 out]
      }
      frame "V4" {
        n549 = shared-variable-write(w1421, w1418, w1420) -> (w1419:refnum<k21>, w1422:errorcluster)  [unwired: 1 in, 1 out]
        n550 = Flush Stream(8:w1422, 11:w1419) -> (0:w1417:errorcluster, 3:w1416:refnum<k21>)  [unwired: 2 in, 1 out]
      }
      frame "FGGA_pump" {
        n551 = shared-variable-write(w1428, w1425, w1427) -> (w1426:refnum<k21>, w1429:errorcluster)  [unwired: 1 in, 1 out]
        n552 = Flush Stream(8:w1429, 11:w1426) -> (0:w1424:errorcluster, 3:w1423:refnum<k21>)  [unwired: 2 in, 1 out]
      }
      frame "Flight Number" {
        n553 = shared-variable-write(w1435, w1432, w1434) -> (w1433:refnum<k21>, w1436:errorcluster)  [unwired: 1 in, 1 out]
        n554 = Flush Stream(8:w1436, 11:w1433) -> (0:w1431:errorcluster, 3:w1430:refnum<k21>)  [unwired: 2 in, 1 out]
      }
      frame "FGGA_restart" {
        n555 = shared-variable-write(w1442, w1439, w1441) -> (w1440:refnum<k21>, w1443:errorcluster)  [unwired: 1 in, 1 out]
        n556 = Flush Stream(8:w1443, 11:w1440) -> (0:w1438:errorcluster, 3:w1437:refnum<k21>)  [unwired: 2 in, 1 out]
      }
      frame "Stop File Write" {
        n557 = shared-variable-write(w1449, w1446, w1448) -> (w1447:refnum<k21>, w1450:errorcluster)  [unwired: 1 in, 1 out]
        n558 = Flush Stream(8:w1450, 11:w1447) -> (0:w1445:errorcluster, 3:w1444:refnum<k21>)  [unwired: 2 in, 1 out]
      }
    }
  }
  "FGGA command sender error out" <- w48
  n559 = Obtain Queue(name (unnamed)="SO2_Command", element data type=w37) -> (queue out=w46:refnum<queue>, error out=w39:errorcluster)  [unwired: 3 in, 1 out]
  n560 = while {
    tunnel: w46 -> [w1454]
    tunnel: w39 -> [w1453]
    tunnel: [w1451] -> _
    stop <- FALSE stop-if-true
    # "SO2 UI Event Handler Loop"
    n561 = event shown="[2] \"SO2 Zeroing\": Value Change" {
      selector: _ -> [_ _ _ _ _ _ _ _ _ _ _ _ _ _ _ _ _ _]
      dyn-events: _ -> [_ _ _ _ _ _ _ _ _ _ _ _ _ _ _ _ _ _]
      timeout: _ -> [_ _ _ _ _ _ _ _ _ _ _ _ _ _ _ _ _ _]
      tunnel: w1454 -> [w1461 w1469 w1502 w1541 w1610 w1617 w1621 w1628 w1635 w1642 w1649 w1656 w1663 w1670 w1677 w1684 w1691 w1698]
      tunnel: w1453 -> [w1460 w1468 w1501 w1540 w1609 w1616 w1620 w1627 w1634 w1641 w1648 w1655 w1662 w1669 w1676 w1683 w1690 w1697]
      tunnel: [w1455 w1467 w1500 _ w1604 w1611 w1619 w1626 w1633 w1640 w1647 w1654 w1661 w1668 w1675 w1682 w1689 w1696] -> w1451
      event "V9": Value Change {
        n562 = event-data() -> ("NewVal"=w1458:bool)  [unwired: 1 in]
        n563 = Bundle(cluster=T4 {"Message"="", "Message Data"=variant} ("Message Cluster"), "Message"="V9", "Message Data"=w1458) -> (w1456:T4)
        n564 = Enqueue Element(queue=w1461, element=w1456, error in (no error)=w1460) -> (error out=w1455:errorcluster)  [unwired: 1 in, 2 out]
      }
      event "SO2 Flush": Value Change {
        n565 = event-data() -> ()  [unwired: 1 in, 1 out]
        n566 = flat-sequence {
          tunnel: w1469 -> [w1477]
          tunnel: w1468 -> [w1476]
          tunnel: [w1472] -> w1466
          tunnel: [w1470] -> w1462
          tunnel: w1466 -> [w1480]
          tunnel: [w1480] -> w1465
          tunnel: [w1478] -> w1463
          tunnel: w1462 -> [w1478]
          tunnel: w1465 -> [w1488]
          tunnel: [w1487] -> w1464
          tunnel: w1463 -> [w1489]
          tunnel: [w1494] -> w1467
          tunnel: w1464 -> [w1494]
          frame #0 {
            w1471 = TRUE ("SO2 Flush")
            n567 = Bundle(cluster=T4 {"Message"="", "Message Data"=variant} ("Message Cluster"), "Message"="V9", "Message Data"=w1471) -> (w1473:T4)
            n568 = local write "V9"(w1471) -> ()
            n569 = Enqueue Element(queue=w1477, element=w1473, error in (no error)=w1476) -> (queue out=w1470:refnum<queue>, error out=w1472:errorcluster)  [unwired: 1 in, 1 out]
          }
          frame #1 {
            n570 = for {
              N: 15 -> [w1484]
              i -> [w1483]
              n571 = Subtract(x=w1484, y=w1483) -> (x-y=w1482:i32)
              n572 = Decrement(x=w1482) -> (x-1=w1481:i32)
              n573 = local write "SO2 Flush\nTime Remain (sec)"(w1481) -> ()
              n574 = Wait (ms)(milliseconds to wait=u32 1000) -> ()  [unwired: 1 out]
            }
          }
          frame #2 {
            w1486 = FALSE
            n575 = Bundle(cluster=T4 {"Message"="", "Message Data"=variant} ("Message Cluster"), "Message"="V9", "Message Data"=w1486) -> (w1490:T4)
            n576 = local write "V9"(w1486) -> ()
            n577 = Enqueue Element(queue=w1489, element=w1490, error in (no error)=w1488) -> (error out=w1487:errorcluster)  [unwired: 1 in, 2 out]
          }
          frame #3 {
            n578 = local write "SO2 Flush"(FALSE ("SO2 Flush")) -> ()
          }
        }
      }
      event "SO2 Zeroing": Value Change {
        n579 = event-data() -> ()  [unwired: 1 in, 1 out]
        n580 = flat-sequence {
          tunnel: w1502 -> [w1510]
          tunnel: w1501 -> [w1509]
          tunnel: [w1505] -> w1499
          tunnel: [w1503] -> w1495
          tunnel: w1499 -> [w1513]
          tunnel: [w1513] -> w1498
          tunnel: [w1511] -> w1496
          tunnel: w1495 -> [w1511]
          tunnel: w1498 -> [w1521]
          tunnel: [w1520] -> w1497
          tunnel: w1496 -> [w1522]
          tunnel: [w1527] -> w1500
          tunnel: w1497 -> [w1527]
          frame #0 {
            w1504 = TRUE ("SO2 Flush")
            n581 = local write "SO2 V6"(w1504) -> ()
            n582 = Bundle(cluster=T4 {"Message"="", "Message Data"=variant} ("Message Cluster"), "Message"="V6", "Message Data"=w1504) -> (w1506:T4)
            n583 = Enqueue Element(queue=w1510, element=w1506, error in (no error)=w1509) -> (queue out=w1503:refnum<queue>, error out=w1505:errorcluster)  [unwired: 1 in, 1 out]
          }
          frame #1 {
            # "10 Mins Count down"
            n584 = for {
              N: 600 -> [w1517]
              i -> [w1516]
              n585 = Subtract(x=w1517, y=w1516) -> (x-y=w1515:i32)
              n586 = Decrement(x=w1515) -> (x-1=w1514:i32)
              n587 = local write "SO2 Zeroing\nTime Remain (sec)"(w1514) -> ()
              n588 = Wait (ms)(milliseconds to wait=u32 1000) -> ()  [unwired: 1 out]
            }
          }
          frame #2 {
            w1519 = FALSE
            n589 = Bundle(cluster=T4 {"Message"="", "Message Data"=variant} ("Message Cluster"), "Message"="V6", "Message Data"=w1519) -> (w1523:T4)
            n590 = local write "SO2 V6"(w1519) -> ()
            n591 = Enqueue Element(queue=w1522, element=w1523, error in (no error)=w1521) -> (error out=w1520:errorcluster)  [unwired: 1 in, 2 out]
          }
          frame #3 {
            n592 = local write "SO2 Zeroing"(FALSE ("SO2 Flush")) -> ()
          }
        }
      }
      event "SO2 CAL": Value Change {
        n593 = event-data() -> ()  [unwired: 1 in, 1 out]
        n594 = flat-sequence {
          tunnel: w1541 -> [w1549]
          tunnel: w1540 -> [w1548]
          tunnel: [w1544] -> w1539
          tunnel: [w1543] -> w1537
          tunnel: w1539 -> [w1553]
          tunnel: [w1552] -> w1538
          tunnel: w1537 -> [w1554]
          tunnel: [w1550] -> w1535
          tunnel: w1538 -> [w1560]
          tunnel: [w1560] -> w1536
          tunnel: w1535 -> [w1558]
          tunnel: [w1558] -> w1534
          tunnel: w1536 -> [w1569]
          tunnel: w1534 -> [w1570]
          tunnel: [w1567] -> w1532
          tunnel: [w1566] -> w1530
          tunnel: [w1575] -> w1533
          tunnel: w1532 -> [w1575]
          tunnel: [w1574] -> w1531
          tunnel: w1530 -> [w1574]
          tunnel: w1533 -> [w1585]
          tunnel: w1531 -> [w1584]
          tunnel: [w1583] -> w1529
          tunnel: [w1582] -> w1528
          tunnel: w1529 -> [w1599]
          tunnel: w1528 -> [w1598]
          frame #0 {
            w1542 = TRUE ("SO2 Flush")
            n595 = Bundle(cluster=T4 {"Message"="", "Message Data"=variant} ("Message Cluster"), "Message"="V9", "Message Data"=w1542) -> (w1545:T4)
            n596 = local write "V9"(w1542) -> ()
            n597 = Enqueue Element(queue=w1549, element=w1545, error in (no error)=w1548) -> (queue out=w1543:refnum<queue>, error out=w1544:errorcluster)  [unwired: 1 in, 1 out]
          }
          frame #1 {
            n598 = local read "MFC_2 User Set Value"() -> (w1551:dbl)
            n599 = local write "MFC_2\nSLPM Value"(w1551) -> ()
            n600 = Bundle(cluster=T4 {"Message"="", "Message Data"=variant} ("Message Cluster"), "Message"="MFC_2", "Message Data"=w1551) -> (w1555:T4)
            n601 = Enqueue Element(queue=w1554, element=w1555, error in (no error)=w1553) -> (queue out=w1550:refnum<queue>, error out=w1552:errorcluster)  [unwired: 1 in, 1 out]
          }
          frame #2 {
            n602 = for {
              N: 45 -> [w1564]
              i -> [w1563]
              n603 = Subtract(x=w1564, y=w1563) -> (x-y=w1562:i32)
              n604 = Decrement(x=w1562) -> (x-1=w1561:i32)
              n605 = local write "SO2 Flush\nTime Remain (sec)"(w1561) -> ()
              n606 = Wait (ms)(milliseconds to wait=u32 1000) -> ()  [unwired: 1 out]
            }
          }
          frame #3 {
            w1568 = TRUE ("SO2 Flush")
            n607 = Bundle(cluster=T4 {"Message"="", "Message Data"=variant} ("Message Cluster"), "Message"="V8", "Message Data"=w1568) -> (w1571:T4)
            n608 = local write "V8"(w1568) -> ()
            n609 = Enqueue Element(queue=w1570, element=w1571, error in (no error)=w1569) -> (queue out=w1567:refnum<queue>, error out=w1566:errorcluster)  [unwired: 1 in, 1 out]
          }
          frame #4 {
            n610 = for {
              N: 60 -> [w1580]
              i -> [w1579]
              n611 = Subtract(x=w1580, y=w1579) -> (x-y=w1578:i32)
              n612 = Decrement(x=w1578) -> (x-1=w1577:i32)
              n613 = local write "SO2 CAL\nTime Remain (sec)"(w1577) -> ()
              n614 = Wait (ms)(milliseconds to wait=u32 1000) -> ()  [unwired: 1 out]
            }
          }
          frame #5 {
            n615 = Cluster To Array(cluster=cluster{"Message":string, "Message 2":string} {"Message"="V8", "Message 2"="V9"}) -> (array=w1587:string[])
            n616 = for {
              tunnel: w1587 -> [w1594] mode=indexing
              tunnel: FALSE ("SO2 Flush") -> [w1593]
              tunnel: w1585 -> [w1592]
              tunnel: w1584 -> [w1591]
              tunnel: [w1590] -> w1583
              tunnel: [w1589] -> w1582
              n617 = Bundle(cluster=T4 {"Message"="", "Message Data"=variant} ("Message Cluster"), "Message"=w1594, "Message Data"=w1593) -> (w1595:T4)
              n618 = Enqueue Element(queue=w1592, element=w1595, error in (no error)=w1591) -> (queue out=w1590:refnum<queue>, error out=w1589:errorcluster)  [unwired: 1 in, 1 out]
            }
          }
          frame #6 {
            w1597 = 0.0 ("MFC_2\nSLPM Value")
            n619 = local write "MFC_2\nSLPM Value"(w1597) -> ()
            n620 = Bundle(cluster=T4 {"Message"="", "Message Data"=variant} ("Message Cluster"), "Message"="MFC_2", "Message Data"=w1597) -> (w1600:T4)
            n621 = Enqueue Element(queue=w1599, element=w1600, error in (no error)=w1598) -> ()  [unwired: 1 in, 3 out]
          }
          frame #7 {
            w1603 = FALSE ("SO2 Flush")
            n622 = local write "SO2 CAL"(w1603) -> ()
            n623 = local write "V9"(w1603) -> ()
            n624 = local write "V8"(w1603) -> ()
          }
        }
      }
      event "MFC_2\nSLPM Value": Value Change {
        n625 = event-data() -> ("NewVal"=w1607:dbl)  [unwired: 1 in]
        n626 = Bundle(cluster=T4 {"Message"="", "Message Data"=variant} ("Message Cluster"), "Message"="MFC_2", "Message Data"=w1607) -> (w1605:T4)
        n627 = Enqueue Element(queue=w1610, element=w1605, error in (no error)=w1609) -> (error out=w1604:errorcluster)  [unwired: 1 in, 2 out]
      }
      event "MFC_3\nSLPM Value": Value Change {
        n628 = event-data() -> ("NewVal"=w1614:dbl)  [unwired: 1 in]
        n629 = Bundle(cluster=T4 {"Message"="", "Message Data"=variant} ("Message Cluster"), "Message"="MFC_3", "Message Data"=w1614) -> (w1612:T4)
        n630 = Enqueue Element(queue=w1617, element=w1612, error in (no error)=w1616) -> (error out=w1611:errorcluster)  [unwired: 1 in, 2 out]
      }
      event "V8": Value Change {
        n631 = event-data() -> ("NewVal"=w1618:bool)  [unwired: 1 in]
        n632 = Bundle(cluster=T4 {"Message"="", "Message Data"=variant} ("Message Cluster"), "Message"="V8", "Message Data"=w1618) -> (w1622:T4)
        n633 = Enqueue Element(queue=w1621, element=w1622, error in (no error)=w1620) -> (error out=w1619:errorcluster)  [unwired: 1 in, 2 out]
      }
      event "SO2 V6": Value Change {
        n634 = event-data() -> ("NewVal"=w1625:bool)  [unwired: 1 in]
        n635 = Bundle(cluster=T4 {"Message"="", "Message Data"=variant} ("Message Cluster"), "Message"="V6", "Message Data"=w1625) -> (w1629:T4)
        n636 = Enqueue Element(queue=w1628, element=w1629, error in (no error)=w1627) -> (error out=w1626:errorcluster)  [unwired: 1 in, 2 out]
      }
      event "Simulate Conc": Value Change {
        n637 = event-data() -> ("NewVal"=w1632:bool)  [unwired: 1 in]
        n638 = Bundle(cluster=T4 {"Message"="", "Message Data"=variant} ("Message Cluster"), "Message"="Simulate Conc", "Message Data"=w1632) -> (w1636:T4)
        n639 = Enqueue Element(queue=w1635, element=w1636, error in (no error)=w1634) -> (error out=w1633:errorcluster)  [unwired: 1 in, 2 out]
      }
      event "SO2 UDP Time Offset": Value Change {
        n640 = event-data() -> ("NewVal"=w1639:i32)  [unwired: 1 in]
        n641 = Bundle(cluster=T4 {"Message"="", "Message Data"=variant} ("Message Cluster"), "Message"="UDP Time Offset", "Message Data"=w1639) -> (w1643:T4)
        n642 = Enqueue Element(queue=w1642, element=w1643, error in (no error)=w1641) -> (error out=w1640:errorcluster)  [unwired: 1 in, 2 out]
      }
      event "Simulate STEL Conc": Value Change {
        n643 = event-data() -> ("NewVal"=w1646:dbl)  [unwired: 1 in]
        n644 = Bundle(cluster=T4 {"Message"="", "Message Data"=variant} ("Message Cluster"), "Message"="Simulate STEL Conc", "Message Data"=w1646) -> (w1650:T4)
        n645 = Enqueue Element(queue=w1649, element=w1650, error in (no error)=w1648) -> (error out=w1647:errorcluster)  [unwired: 1 in, 2 out]
      }
      event "Simulate TWA Conc": Value Change {
        n646 = event-data() -> ("NewVal"=w1653:dbl)  [unwired: 1 in]
        n647 = Bundle(cluster=T4 {"Message"="", "Message Data"=variant} ("Message Cluster"), "Message"="Simulate TWA Conc", "Message Data"=w1653) -> (w1657:T4)
        n648 = Enqueue Element(queue=w1656, element=w1657, error in (no error)=w1655) -> (error out=w1654:errorcluster)  [unwired: 1 in, 2 out]
      }
      event "10mins STEL Limit": Value Change {
        n649 = event-data() -> ("NewVal"=w1660:i32)  [unwired: 1 in]
        n650 = Bundle(cluster=T4 {"Message"="", "Message Data"=variant} ("Message Cluster"), "Message"="10mins STEL Limit", "Message Data"=w1660) -> (w1664:T4)
        n651 = Enqueue Element(queue=w1663, element=w1664, error in (no error)=w1662) -> (error out=w1661:errorcluster)  [unwired: 1 in, 2 out]
      }
      event "8hr TWA Limit": Value Change {
        n652 = event-data() -> ("NewVal"=w1667:i32)  [unwired: 1 in]
        n653 = Bundle(cluster=T4 {"Message"="", "Message Data"=variant} ("Message Cluster"), "Message"="8hr TWA Limit", "Message Data"=w1667) -> (w1671:T4)
        n654 = Enqueue Element(queue=w1670, element=w1671, error in (no error)=w1669) -> (error out=w1668:errorcluster)  [unwired: 1 in, 2 out]
      }
      event "SO2 Offset": Value Change {
        n655 = event-data() -> ("NewVal"=w1674:dbl)  [unwired: 1 in]
        n656 = Bundle(cluster=T4 {"Message"="", "Message Data"=variant} ("Message Cluster"), "Message"="Offset", "Message Data"=w1674) -> (w1678:T4)
        n657 = Enqueue Element(queue=w1677, element=w1678, error in (no error)=w1676) -> (error out=w1675:errorcluster)  [unwired: 1 in, 2 out]
      }
      event "SO2 Slope": Value Change {
        n658 = event-data() -> ("NewVal"=w1681:dbl)  [unwired: 1 in]
        n659 = Bundle(cluster=T4 {"Message"="", "Message Data"=variant} ("Message Cluster"), "Message"="Slope", "Message Data"=w1681) -> (w1685:T4)
        n660 = Enqueue Element(queue=w1684, element=w1685, error in (no error)=w1683) -> (error out=w1682:errorcluster)  [unwired: 1 in, 2 out]
      }
      event "Confirm Flight Number": Value Change {
        n661 = event-data() -> ()  [unwired: 1 in, 6 out]
        n662 = local read "Flight Number"() -> (w1688:string)
        n663 = Bundle(cluster=T4 {"Message"="", "Message Data"=variant} ("Message Cluster"), "Message"="Flight Number", "Message Data"=w1688) -> (w1692:T4)
        n664 = Enqueue Element(queue=w1691, element=w1692, error in (no error)=w1690) -> (error out=w1689:errorcluster)  [unwired: 1 in, 2 out]
      }
      event "cRIO File IO Stop\n(USB Flash Drive Unmount)": Value Change {
        n665 = event-data() -> ("NewVal"=w1695:bool)  [unwired: 1 in]
        n666 = Bundle(cluster=T4 {"Message"="", "Message Data"=variant} ("Message Cluster"), "Message"="Stop File Write", "Message Data"=w1695) -> (w1699:T4)
        n667 = Enqueue Element(queue=w1698, element=w1699, error in (no error)=w1697) -> (error out=w1696:errorcluster)  [unwired: 1 in, 2 out]
      }
    }
    "SO2 Event error out" <- w1451
  }
  n668 = Create Network Stream Writer Endpoint(6:w43, 7:10 ("writer buffer size"), 9:w37, 10:"//192.168.101.17/command/reader/SO2" ("reader url"), 11:"/command/writer/SO2" ("writer name")) -> (0:w42:errorcluster, 3:w41:refnum<k21>)  [unwired: 2 in]
  n669 = while {
    tunnel: w46 -> [w1709]
    shift-right: [w1704] -> _
    shift-left: w41 -> [w1706]
    shift-right: [w1702] -> w38
    shift-left: w42 -> [w1708]
    tunnel: w39 -> [w1703]
    stop <- w1702 stop-if-true
    # "SO2 UI Command Sender"
    n670 = Dequeue Element(queue=w1709, error in (no error)=w1703) -> (element=w1705:T4)  [unwired: 1 in, 3 out]
    n671 = Unbundle By Name(w1705) -> ("Message"=w1707:string)
    n672 = case shown="\"UDP Time Offset\"" w1707 {
      tunnel: w1708 -> [w1710 w1714 w1721 w1728 w1735 w1742 w1749 w1756 w1763 w1770 w1777 w1784 w1791 w1798 w1805 w1812]
      tunnel: w1706 -> [w1711 w1717 w1724 w1731 w1738 w1745 w1752 w1759 w1766 w1773 w1780 w1787 w1794 w1801 w1808 w1815]
      tunnel: w1705 -> [_ w1716 w1723 w1730 w1737 w1744 w1751 w1758 w1765 w1772 w1779 w1786 w1793 w1800 w1807 w1814]
      tunnel: [w1710 w1713 w1720 w1727 w1734 w1741 w1748 w1755 w1762 w1769 w1776 w1783 w1790 w1797 w1804 w1811] -> w1702
      tunnel: [w1711 w1712 w1719 w1726 w1733 w1740 w1747 w1754 w1761 w1768 w1775 w1782 w1789 w1796 w1803 w1810] -> w1704
      frame "False", Default {
      }
      frame "V9" {
        n673 = shared-variable-write(w1717, w1714, w1716) -> (w1715:refnum<k21>, w1718:errorcluster)  [unwired: 1 in, 1 out]
        n674 = Flush Stream(8:w1718, 11:w1715) -> (0:w1713:errorcluster, 3:w1712:refnum<k21>)  [unwired: 2 in, 1 out]
      }
      frame "MFC_2" {
        n675 = shared-variable-write(w1724, w1721, w1723) -> (w1722:refnum<k21>, w1725:errorcluster)  [unwired: 1 in, 1 out]
        n676 = Flush Stream(8:w1725, 11:w1722) -> (0:w1720:errorcluster, 3:w1719:refnum<k21>)  [unwired: 2 in, 1 out]
      }
      frame "MFC_3" {
        n677 = shared-variable-write(w1731, w1728, w1730) -> (w1729:refnum<k21>, w1732:errorcluster)  [unwired: 1 in, 1 out]
        n678 = Flush Stream(8:w1732, 11:w1729) -> (0:w1727:errorcluster, 3:w1726:refnum<k21>)  [unwired: 2 in, 1 out]
      }
      frame "V6" {
        n679 = shared-variable-write(w1738, w1735, w1737) -> (w1736:refnum<k21>, w1739:errorcluster)  [unwired: 1 in, 1 out]
        n680 = Flush Stream(8:w1739, 11:w1736) -> (0:w1734:errorcluster, 3:w1733:refnum<k21>)  [unwired: 2 in, 1 out]
      }
      frame "Simulate Conc" {
        n681 = shared-variable-write(w1745, w1742, w1744) -> (w1743:refnum<k21>, w1746:errorcluster)  [unwired: 1 in, 1 out]
        n682 = Flush Stream(8:w1746, 11:w1743) -> (0:w1741:errorcluster, 3:w1740:refnum<k21>)  [unwired: 2 in, 1 out]
      }
      frame "Simulate STEL Conc" {
        n683 = shared-variable-write(w1752, w1749, w1751) -> (w1750:refnum<k21>, w1753:errorcluster)  [unwired: 1 in, 1 out]
        n684 = Flush Stream(8:w1753, 11:w1750) -> (0:w1748:errorcluster, 3:w1747:refnum<k21>)  [unwired: 2 in, 1 out]
      }
      frame "Simulate TWA Conc" {
        n685 = shared-variable-write(w1759, w1756, w1758) -> (w1757:refnum<k21>, w1760:errorcluster)  [unwired: 1 in, 1 out]
        n686 = Flush Stream(8:w1760, 11:w1757) -> (0:w1755:errorcluster, 3:w1754:refnum<k21>)  [unwired: 2 in, 1 out]
      }
      frame "10mins STEL Limit" {
        n687 = shared-variable-write(w1766, w1763, w1765) -> (w1764:refnum<k21>, w1767:errorcluster)  [unwired: 1 in, 1 out]
        n688 = Flush Stream(8:w1767, 11:w1764) -> (0:w1762:errorcluster, 3:w1761:refnum<k21>)  [unwired: 2 in, 1 out]
      }
      frame "8hr TWA Limit" {
        n689 = shared-variable-write(w1773, w1770, w1772) -> (w1771:refnum<k21>, w1774:errorcluster)  [unwired: 1 in, 1 out]
        n690 = Flush Stream(8:w1774, 11:w1771) -> (0:w1769:errorcluster, 3:w1768:refnum<k21>)  [unwired: 2 in, 1 out]
      }
      frame "Offset" {
        n691 = shared-variable-write(w1780, w1777, w1779) -> (w1778:refnum<k21>, w1781:errorcluster)  [unwired: 1 in, 1 out]
        n692 = Flush Stream(8:w1781, 11:w1778) -> (0:w1776:errorcluster, 3:w1775:refnum<k21>)  [unwired: 2 in, 1 out]
      }
      frame "Slope" {
        n693 = shared-variable-write(w1787, w1784, w1786) -> (w1785:refnum<k21>, w1788:errorcluster)  [unwired: 1 in, 1 out]
        n694 = Flush Stream(8:w1788, 11:w1785) -> (0:w1783:errorcluster, 3:w1782:refnum<k21>)  [unwired: 2 in, 1 out]
      }
      frame "Flight Number" {
        n695 = shared-variable-write(w1794, w1791, w1793) -> (w1792:refnum<k21>, w1795:errorcluster)  [unwired: 1 in, 1 out]
        n696 = Flush Stream(8:w1795, 11:w1792) -> (0:w1790:errorcluster, 3:w1789:refnum<k21>)  [unwired: 2 in, 1 out]
      }
      frame "Stop File Write" {
        n697 = shared-variable-write(w1801, w1798, w1800) -> (w1799:refnum<k21>, w1802:errorcluster)  [unwired: 1 in, 1 out]
        n698 = Flush Stream(8:w1802, 11:w1799) -> (0:w1797:errorcluster, 3:w1796:refnum<k21>)  [unwired: 2 in, 1 out]
      }
      frame "UDP Time Offset" {
        n699 = shared-variable-write(w1808, w1805, w1807) -> (w1806:refnum<k21>, w1809:errorcluster)  [unwired: 1 in, 1 out]
        n700 = Flush Stream(8:w1809, 11:w1806) -> (0:w1804:errorcluster, 3:w1803:refnum<k21>)  [unwired: 2 in, 1 out]
      }
      frame "V8" {
        n701 = shared-variable-write(w1815, w1812, w1814) -> (w1813:refnum<k21>, w1816:errorcluster)  [unwired: 1 in, 1 out]
        n702 = Flush Stream(8:w1816, 11:w1813) -> (0:w1811:errorcluster, 3:w1810:refnum<k21>)  [unwired: 2 in, 1 out]
      }
    }
  }
  "SO2 command sender error out" <- w38
  n703 = Obtain Queue(name (unnamed)="TEi43c_Command", element data type=w26) -> (queue out=w35:refnum<queue>, error out=w28:errorcluster)  [unwired: 3 in, 1 out]
  n704 = Create Network Stream Writer Endpoint(6:w32, 7:10 ("writer buffer size"), 9:w26, 10:"//192.168.101.17/command/reader/TEi43c" ("reader url"), 11:"/command/writer/TEi43c" ("writer name")) -> (0:w31:errorcluster, 3:w30:refnum<k21>)  [unwired: 2 in]
  n705 = while {
    tunnel: w35 -> [w1820]
    tunnel: w28 -> [w1819]
    tunnel: [w1817] -> _
    stop <- FALSE stop-if-true
    # "TEi43c Ozone UI Event Handler Loop"
    n706 = event shown="[0] \"Ozone Zeroing\": Value Change" {
      selector: _ -> [_ _ _ _ _]
      dyn-events: _ -> [_ _ _ _ _]
      timeout: _ -> [_ _ _ _ _]
      tunnel: w1820 -> [w1828 w1856 w1864 w1871 w1878]
      tunnel: w1819 -> [w1827 w1855 w1863 w1870 w1877]
      tunnel: [w1826 w1854 w1862 w1869 w1876] -> w1817
      event "Ozone Zeroing": Value Change {
        n707 = event-data() -> ()  [unwired: 1 in, 6 out]
        n708 = flat-sequence {
          tunnel: w1828 -> [w1833]
          tunnel: w1827 -> [w1832]
          tunnel: [w1831] -> w1825
          tunnel: [w1829] -> w1821
          tunnel: w1825 -> [w1839]
          tunnel: [w1839] -> w1824
          tunnel: [w1837] -> w1822
          tunnel: w1821 -> [w1837]
          tunnel: w1824 -> [w1847]
          tunnel: [w1846] -> w1823
          tunnel: w1822 -> [w1848]
          tunnel: [w1853] -> w1826
          tunnel: w1823 -> [w1853]
          frame #0 {
            w1830 = TRUE
            n709 = local write "Ozone V6"(w1830) -> ()
            n710 = Bundle(cluster=T4 {"Message"="", "Message Data"=variant} ("Message Cluster"), "Message"="V6", "Message Data"=w1830) -> (w1834:T4)
            n711 = Enqueue Element(queue=w1833, element=w1834, error in (no error)=w1832) -> (queue out=w1829:refnum<queue>, error out=w1831:errorcluster)  [unwired: 1 in, 1 out]
          }
          frame #1 {
            # "10 Mins Count down"
            n712 = for {
              N: 600 -> [w1843]
              i -> [w1842]
              n713 = Subtract(x=w1843, y=w1842) -> (x-y=w1841:i32)
              n714 = Decrement(x=w1841) -> (x-1=→"Ozone Zeroing\nTime Remain (sec)":i32)
              n715 = Wait (ms)(milliseconds to wait=u32 1000) -> ()  [unwired: 1 out]
            }
          }
          frame #2 {
            w1845 = FALSE
            n716 = local write "Ozone V6"(w1845) -> ()
            n717 = Bundle(cluster=T4 {"Message"="", "Message Data"=variant} ("Message Cluster"), "Message"="V6", "Message Data"=w1845) -> (w1849:T4)
            n718 = Enqueue Element(queue=w1848, element=w1849, error in (no error)=w1847) -> (error out=w1846:errorcluster)  [unwired: 1 in, 2 out]
          }
          frame #3 {
            n719 = local write "Ozone Zeroing"(FALSE ("Ozone Zeroing")) -> ()
          }
        }
      }
      event "Ozone V6": Value Change {
        n720 = event-data() -> ("NewVal"=w1857:bool)  [unwired: 1 in]
        n721 = Bundle(cluster=T4 {"Message"="", "Message Data"=variant} ("Message Cluster"), "Message"="V6", "Message Data"=w1857) -> (w1858:T4)
        n722 = Enqueue Element(queue=w1856, element=w1858, error in (no error)=w1855) -> (error out=w1854:errorcluster)  [unwired: 1 in, 2 out]
      }
      event "cRIO File IO Stop\n(USB Flash Drive Unmount)": Value Change {
        n723 = event-data() -> ("NewVal"=w1861:bool)  [unwired: 1 in]
        n724 = Bundle(cluster=T4 {"Message"="", "Message Data"=variant} ("Message Cluster"), "Message"="Stop File Write", "Message Data"=w1861) -> (w1865:T4)
        n725 = Enqueue Element(queue=w1864, element=w1865, error in (no error)=w1863) -> (error out=w1862:errorcluster)  [unwired: 1 in, 2 out]
      }
      event "Ozone UDP Time Offset": Value Change {
        n726 = event-data() -> ("NewVal"=w1868:i32)  [unwired: 1 in]
        n727 = Bundle(cluster=T4 {"Message"="", "Message Data"=variant} ("Message Cluster"), "Message"="UDP Time Offset", "Message Data"=w1868) -> (w1872:T4)
        n728 = Enqueue Element(queue=w1871, element=w1872, error in (no error)=w1870) -> (error out=w1869:errorcluster)  [unwired: 1 in, 2 out]
      }
      event "Confirm Flight Number": Value Change {
        n729 = event-data() -> ()  [unwired: 1 in, 5 out]
        n730 = local read "Flight Number"() -> (w1875:string)
        n731 = Bundle(cluster=T4 {"Message"="", "Message Data"=variant} ("Message Cluster"), "Message"="Flight Number", "Message Data"=w1875) -> (w1879:T4)
        n732 = Enqueue Element(queue=w1878, element=w1879, error in (no error)=w1877) -> (error out=w1876:errorcluster)  [unwired: 1 in, 2 out]
      }
    }
    "Ozone Event error out" <- w1817
  }
  n733 = while {
    tunnel: w35 -> [w1889]
    shift-right: [w1884] -> _
    shift-left: w30 -> [w1886]
    shift-right: [w1882] -> w27
    shift-left: w31 -> [w1888]
    tunnel: w28 -> [w1883]
    stop <- w1882 stop-if-true
    # "TEi43c Ozone UI Command Sender"
    n734 = Dequeue Element(queue=w1889, error in (no error)=w1883) -> (element=w1885:T4)  [unwired: 1 in, 3 out]
    n735 = Unbundle By Name(w1885) -> ("Message"=w1887:string)
    n736 = case shown="\"UDP Time Offset\"" w1887 {
      tunnel: w1888 -> [w1890 w1894 w1901 w1908 w1915]
      tunnel: w1886 -> [w1891 w1897 w1904 w1911 w1918]
      tunnel: w1885 -> [_ w1896 w1903 w1910 w1917]
      tunnel: [w1890 w1893 w1900 w1907 w1914] -> w1882
      tunnel: [w1891 w1892 w1899 w1906 w1913] -> w1884
      frame "False", Default {
      }
      frame "V6" {
        n737 = shared-variable-write(w1897, w1894, w1896) -> (w1895:refnum<k21>, w1898:errorcluster)  [unwired: 1 in, 1 out]
        n738 = Flush Stream(8:w1898, 11:w1895) -> (0:w1893:errorcluster, 3:w1892:refnum<k21>)  [unwired: 2 in, 1 out]
      }
      frame "Stop File Write" {
        n739 = shared-variable-write(w1904, w1901, w1903) -> (w1902:refnum<k21>, w1905:errorcluster)  [unwired: 1 in, 1 out]
        n740 = Flush Stream(8:w1905, 11:w1902) -> (0:w1900:errorcluster, 3:w1899:refnum<k21>)  [unwired: 2 in, 1 out]
      }
      frame "Flight Number" {
        n741 = shared-variable-write(w1911, w1908, w1910) -> (w1909:refnum<k21>, w1912:errorcluster)  [unwired: 1 in, 1 out]
        n742 = Flush Stream(8:w1912, 11:w1909) -> (0:w1907:errorcluster, 3:w1906:refnum<k21>)  [unwired: 2 in, 1 out]
      }
      frame "UDP Time Offset" {
        n743 = shared-variable-write(w1918, w1915, w1917) -> (w1916:refnum<k21>, w1919:errorcluster)  [unwired: 1 in, 1 out]
        n744 = Flush Stream(8:w1919, 11:w1916) -> (0:w1914:errorcluster, 3:w1913:refnum<k21>)  [unwired: 2 in, 1 out]
      }
    }
  }
  "Ozone command sender error out" <- w27
  n745 = Obtain Queue(name (unnamed)="2BOzone_Command", element data type=w14) -> (queue out=w23:refnum<queue>, error out=w16:errorcluster)  [unwired: 3 in, 1 out]
  n746 = Create Network Stream Writer Endpoint(6:w20, 7:10 ("writer buffer size"), 9:w14, 10:"//192.168.101.17/command/reader/2BOzone" ("reader url"), 11:"/command/writer/2BOzone" ("writer name")) -> (0:w19:errorcluster, 3:w18:refnum<k21>)  [unwired: 2 in]
  n747 = while {
    tunnel: w23 -> [w1923]
    tunnel: w16 -> [w1922]
    tunnel: [w1920] -> _
    stop <- FALSE stop-if-true
    # "2BOzone UI Event Handler Loop"
    n748 = event shown="[7] \"Confirm Flight Number\": Value Change" {
      selector: _ -> [_ _ _ _ _ _ _ _]
      dyn-events: _ -> [_ _ _ _ _ _ _ _]
      timeout: _ -> [_ _ _ _ _ _ _ _]
      tunnel: w1923 -> [w1927 w1934 w1941 w1948 w1955 w1962 w1969 w1976]
      tunnel: w1922 -> [w1926 w1933 w1940 w1947 w1954 w1961 w1968 w1975]
      tunnel: [w1925 w1932 w1939 w1946 w1953 w1960 w1967 w1974] -> w1920
      event "Ambient = OFF\nCabin = ON": Value Change {
        n749 = event-data() -> ("NewVal"=w1924:bool)  [unwired: 1 in]
        n750 = Bundle(cluster=T4 {"Message"="", "Message Data"=variant} ("Message Cluster"), "Message"="Ambient/Cabin", "Message Data"=w1924) -> (w1928:T4)
        n751 = Enqueue Element(queue=w1927, element=w1928, error in (no error)=w1926) -> (error out=w1925:errorcluster)  [unwired: 1 in, 2 out]
      }
      event "Simulate 2B Conc": Value Change {
        n752 = event-data() -> ("NewVal"=w1931:bool)  [unwired: 1 in]
        n753 = Bundle(cluster=T4 {"Message"="", "Message Data"=variant} ("Message Cluster"), "Message"="Simulate_conc", "Message Data"=w1931) -> (w1935:T4)
        n754 = Enqueue Element(queue=w1934, element=w1935, error in (no error)=w1933) -> (error out=w1932:errorcluster)  [unwired: 1 in, 2 out]
      }
      event "Simulate Inst Conc": Value Change {
        n755 = event-data() -> ("NewVal"=w1938:i32)  [unwired: 1 in]
        n756 = Bundle(cluster=T4 {"Message"="", "Message Data"=variant} ("Message Cluster"), "Message"="Simulate_inst_conc", "Message Data"=w1938) -> (w1942:T4)
        n757 = Enqueue Element(queue=w1941, element=w1942, error in (no error)=w1940) -> (error out=w1939:errorcluster)  [unwired: 1 in, 2 out]
      }
      event "Inst_alm_thresh": Value Change {
        n758 = event-data() -> ("NewVal"=w1945:i32)  [unwired: 1 in]
        n759 = Bundle(cluster=T4 {"Message"="", "Message Data"=variant} ("Message Cluster"), "Message"="Inst_alm_thresh", "Message Data"=w1945) -> (w1949:T4)
        n760 = Enqueue Element(queue=w1948, element=w1949, error in (no error)=w1947) -> (error out=w1946:errorcluster)  [unwired: 1 in, 2 out]
      }
      event "3hr_alm_thresh": Value Change {
        n761 = event-data() -> ("NewVal"=w1952:i32)  [unwired: 1 in]
        n762 = Bundle(cluster=T4 {"Message"="", "Message Data"=variant} ("Message Cluster"), "Message"="3hr_alm_thresh", "Message Data"=w1952) -> (w1956:T4)
        n763 = Enqueue Element(queue=w1955, element=w1956, error in (no error)=w1954) -> (error out=w1953:errorcluster)  [unwired: 1 in, 2 out]
      }
      event "Simulate 3hr Average Conc": Value Change {
        n764 = event-data() -> ("NewVal"=w1959:dbl)  [unwired: 1 in]
        n765 = Bundle(cluster=T4 {"Message"="", "Message Data"=variant} ("Message Cluster"), "Message"="Simulate_3hr_av_conc", "Message Data"=w1959) -> (w1963:T4)
        n766 = Enqueue Element(queue=w1962, element=w1963, error in (no error)=w1961) -> (error out=w1960:errorcluster)  [unwired: 1 in, 2 out]
      }
      event "cRIO File IO Stop\n(USB Flash Drive Unmount)": Value Change {
        n767 = event-data() -> ("NewVal"=w1966:bool)  [unwired: 1 in]
        n768 = Bundle(cluster=T4 {"Message"="", "Message Data"=variant} ("Message Cluster"), "Message"="Stop File Write", "Message Data"=w1966) -> (w1970:T4)
        n769 = Enqueue Element(queue=w1969, element=w1970, error in (no error)=w1968) -> (error out=w1967:errorcluster)  [unwired: 1 in, 2 out]
      }
      event "Confirm Flight Number": Value Change {
        n770 = event-data() -> ()  [unwired: 1 in, 5 out]
        n771 = local read "Flight Number"() -> (w1973:string)
        n772 = Bundle(cluster=T4 {"Message"="", "Message Data"=variant} ("Message Cluster"), "Message"="Flight Number", "Message Data"=w1973) -> (w1977:T4)
        n773 = Enqueue Element(queue=w1976, element=w1977, error in (no error)=w1975) -> (error out=w1974:errorcluster)  [unwired: 1 in, 2 out]
      }
    }
    "2BOzone Event error out" <- w1920
  }
  n774 = while {
    tunnel: w23 -> [w1987]
    shift-right: [w1982] -> _
    shift-left: w18 -> [w1984]
    shift-right: [w1980] -> w15
    shift-left: w19 -> [w1986]
    tunnel: w16 -> [w1981]
    stop <- w1980 stop-if-true
    # "2BOzone UI Command Sender"
    n775 = Dequeue Element(queue=w1987, error in (no error)=w1981) -> (element=w1983:T4)  [unwired: 1 in, 3 out]
    n776 = Unbundle By Name(w1983) -> ("Message"=w1985:string)
    n777 = case shown="\"3hr_alm_thresh\"" w1985 {
      tunnel: w1986 -> [w1988 w1992 w1999 w2006 w2013 w2020 w2027 w2034 w2041]
      tunnel: w1984 -> [w1989 w1995 w2002 w2009 w2016 w2023 w2030 w2037 w2044]
      tunnel: w1983 -> [_ w1994 w2001 w2008 w2015 w2022 w2029 w2036 w2043]
      tunnel: [w1988 w1991 w1998 w2005 w2012 w2019 w2026 w2033 w2040] -> w1980
      tunnel: [w1989 w1990 w1997 w2004 w2011 w2018 w2025 w2032 w2039] -> w1982
      frame "False", Default {
      }
      frame "Ambient/Cabin" {
        n778 = shared-variable-write(w1995, w1992, w1994) -> (w1993:refnum<k21>, w1996:errorcluster)  [unwired: 1 in, 1 out]
        n779 = Flush Stream(8:w1996, 11:w1993) -> (0:w1991:errorcluster, 3:w1990:refnum<k21>)  [unwired: 2 in, 1 out]
      }
      frame "Simulate_conc" {
        n780 = shared-variable-write(w2002, w1999, w2001) -> (w2000:refnum<k21>, w2003:errorcluster)  [unwired: 1 in, 1 out]
        n781 = Flush Stream(8:w2003, 11:w2000) -> (0:w1998:errorcluster, 3:w1997:refnum<k21>)  [unwired: 2 in, 1 out]
      }
      frame "Simulate_inst_conc" {
        n782 = shared-variable-write(w2009, w2006, w2008) -> (w2007:refnum<k21>, w2010:errorcluster)  [unwired: 1 in, 1 out]
        n783 = Flush Stream(8:w2010, 11:w2007) -> (0:w2005:errorcluster, 3:w2004:refnum<k21>)  [unwired: 2 in, 1 out]
      }
      frame "Inst_alm_thresh" {
        n784 = shared-variable-write(w2016, w2013, w2015) -> (w2014:refnum<k21>, w2017:errorcluster)  [unwired: 1 in, 1 out]
        n785 = Flush Stream(8:w2017, 11:w2014) -> (0:w2012:errorcluster, 3:w2011:refnum<k21>)  [unwired: 2 in, 1 out]
      }
      frame "3hr_alm_thresh" {
        n786 = shared-variable-write(w2023, w2020, w2022) -> (w2021:refnum<k21>, w2024:errorcluster)  [unwired: 1 in, 1 out]
        n787 = Flush Stream(8:w2024, 11:w2021) -> (0:w2019:errorcluster, 3:w2018:refnum<k21>)  [unwired: 2 in, 1 out]
      }
      frame "Simulate_3hr_av_conc" {
        n788 = shared-variable-write(w2030, w2027, w2029) -> (w2028:refnum<k21>, w2031:errorcluster)  [unwired: 1 in, 1 out]
        n789 = Flush Stream(8:w2031, 11:w2028) -> (0:w2026:errorcluster, 3:w2025:refnum<k21>)  [unwired: 2 in, 1 out]
      }
      frame "Stop File Write" {
        n790 = shared-variable-write(w2037, w2034, w2036) -> (w2035:refnum<k21>, w2038:errorcluster)  [unwired: 1 in, 1 out]
        n791 = Flush Stream(8:w2038, 11:w2035) -> (0:w2033:errorcluster, 3:w2032:refnum<k21>)  [unwired: 2 in, 1 out]
      }
      frame "Flight Number" {
        n792 = shared-variable-write(w2044, w2041, w2043) -> (w2042:refnum<k21>, w2045:errorcluster)  [unwired: 1 in, 1 out]
        n793 = Flush Stream(8:w2045, 11:w2042) -> (0:w2040:errorcluster, 3:w2039:refnum<k21>)  [unwired: 2 in, 1 out]
      }
    }
  }
  "2BOzone command sender error out" <- w15
